vi "Main.vi"() -> ()   [LabVIEW 2017]
uses:
  type defs/states.ctl
  <vilib>/myRIO/Express VI/Onboard Devices/LED/LED Express VI.xnode
  <vilib>/myRIO/Instrument Drivers/Onboard IO/DIO/vis/Write.vi
  <vilib>/myRIO/Instrument Drivers/Onboard IO/DIO/DIO.lvlib
  <vilib>/myRIO/Common/Instrument Driver Framework/myRIO v1.0/DIO/typedefs/DIO Channels Enum.ctl
  <vilib>/myRIO/Common/Instrument Driver Framework/myRIO v1.0/DIO/typedefs/DIO Channels List.ctl
  <vilib>/myRIO/Common/Instrument Driver Framework/Utilities/typedefs/Generic FPGA Reference.ctl
  <vilib>/myRIO/Common/Instrument Driver Framework/Utilities/typedefs/myRIO v1.0 Reference.ctl
  <vilib>/myRIO/Common/Instrument Driver Framework/Utilities/typedefs/Hardware Version Enum.ctl
  <vilib>/myRIO/Common/Instrument Driver Framework/Utilities/typedefs/myRIO Generic Hardware Reference.ctl
  <vilib>/myRIO/Instrument Drivers/Onboard IO/DIO/typedefs/DIO Reference.ctl
  <vilib>/myRIO/Instrument Drivers/Onboard IO/DIO/vis/myRIO DIO Open.xnode
  <vilib>/myRIO/Common/Instrument Driver Framework/Utilities/vis/Is FPGA Ref Available.vi
  <vilib>/myRIO/Common/Instrument Driver Framework/myRIO v1.0/DIO/vis/myRIO v1.1 Open DIO.vi
  <vilib>/userdefined/High Color/nirio_resource_hc.ctl
  <vilib>/myRIO/Express VI/Onboard Devices/Button/Button Express VI.xnode
  type defs/task.ctl
  <vilib>/myRIO/Instrument Drivers/Onboard IO/PWM/typedefs/PWM Configuration.ctl
  <vilib>/myRIO/Instrument Drivers/Onboard IO/PWM/PWM.lvlib
  <vilib>/myRIO/Common/Instrument Driver Framework/myRIO v1.0/PWM/typedefs/PWM Channels Enum.ctl
  <vilib>/myRIO/Instrument Drivers/Onboard IO/PWM/typedefs/PWM Reference.ctl
  <vilib>/myRIO/Common/Instrument Driver Framework/myRIO v1.0/PWM/vis/myRIO v1.1 Open PWM.vi
  <vilib>/myRIO/Instrument Drivers/Onboard IO/PWM/vis/myRIO PWM Open.xnode
  <vilib>/myRIO/Express VI/Onboard IO/PWM/PWM Express VI.xnode
  <vilib>/myRIO/Express VI/Onboard IO/DO/DO Express VI.xnode
  <vilib>/myRIO/Instrument Drivers/Utilities/Utilities.lvlib
  type defs/data.ctl
  <vilib>/vision/Image Controls.llb/IMAQ Image.ctl
  <vilib>/vision/NI_Vision_Development_Module.lvlib
  <vilib>/myRIO/Instrument Drivers/Onboard IO/I2C/I2C.lvlib
  <vilib>/myRIO/Instrument Drivers/Onboard IO/Encoder/Encoder.lvlib
  <vilib>/myRIO/Common/Instrument Driver Framework/myRIO v1.0/Encoder/typedefs/Encoder Signal Mode.ctl
  type defs/action buttons.ctl
  <vilib>/vision/driver/NI_Vision_Acquisition_Software.lvlib
  <vilib>/userdefined/High Color/IMAQdx.ctl
  <vilib>/myRIO/Instrument Drivers/Onboard IO/I2C/vis/myRIO I2C Open.xnode
  <vilib>/myRIO/Instrument Drivers/Onboard IO/I2C/typedefs/I2C Reference.ctl
  <vilib>/myRIO/Instrument Drivers/Onboard IO/I2C/typedefs/I2C Configuration.ctl
  <vilib>/myRIO/Instrument Drivers/Onboard IO/I2C/typedefs/I2C Transfer Rate.ctl
  <vilib>/myRIO/Common/Instrument Driver Framework/myRIO v1.0/I2C/typedefs/I2C Channels Enum.ctl
  <vilib>/myRIO/Common/Instrument Driver Framework/myRIO v1.0/I2C/vis/myRIO v1.1 Open I2C.vi
  type defs/mode buttons.ctl
  <vilib>/vision/Pattern Matching.llb/IMAQ GM Match Report.ctl
panel:
  out "State":T1(ring)
  in  "BackStates":enum16{"0", "1", "2", "3", "4", "5", "6", ""}(ring)
  in  "At Def pos":bool
  out "Grabbed":bool
  in  "error in":errorcluster
  out "error out 4":errorcluster
  out "error out 3":errorcluster
  out "error out 2":errorcluster
  in  "Def PWM":dbl=0.5
  out "Found Right Ball":bool=TRUE
  out "FT_G_enc":i32[](array[numeric])
  out "FT_M_enc":i32[](array[numeric])
  out "FT_Right_enc":i32[](array[numeric])
  out "FT_Left_enc":i32[](array[numeric])
  out "FT_Angles":dbl[](array[numeric])
  out "Dots of States":i32[][](array[numeric])
  in  "States in total":i32
  in  "(auto) States":T2(ring)
  out "G_enc":i32[](array[numeric])
  out "M_enc":i32[](array[numeric])
  out "Right_enc":i32[](array[numeric])
  out "Left_enc":i32[](array[numeric])
  out "Angles":dbl[](array[numeric])
  in  "Dots in total":i32
  in  "CurDot":T3(ring)
  out "(auto) balls counter":i32
  out "distance to the side":u32
  out "value Z 2":ext
  out "value Z":ext
  in  ",ctl num":i32
  in  ".Task":enum16{"Def", "<mod>[P]+tnl ", "(auto)"}(ring)
  out "Pattern classes":i32[](array[numeric])
  in  "5":i32
  in  "4":i32
  in  "3":i32
  in  "1":i32
  in  "2":i32
  out "5b":bool
  out "4b":bool
  out "3b":bool
  out "2b":bool
  out "1b":bool
  out "Color classes":i32[](array[numeric])
  in  "Next step":bool
  in  "ball = pattern?":bool
  out "error out":errorcluster
  in  "Tab Control":enum32{"Motors", "Ball", "Pattern", "Camera"}(tab)
  in  "Left+":bool
  in  "Left-":bool
  in  "Right+":bool
  in  "Right-":bool
  in  "G-":bool
  in  "G+":bool
  in  "M+":bool
  in  "M-":bool
  in  "M_PWM":dbl=0.4
  in  "L_PWM":dbl=0.5
  in  "R_PWM":dbl=0.5
  in  "Reset M_enc":bool
  out "M_enc_value":i32
  in  "Reset G_enc":bool
  out "G_enc_value":i32
  in  "G_PWM":dbl=0.4
  in  "M_UB_Align":i32=-800
  in  "G_UB_Align":i32
  in  "M_UB_grab":i32=-800
  in  "G_UB_grab":i32=-500
  in  "Manip state":enum16{"Align", "Grab", "Release", "PickUp"}(ring)
  in  "Reset L_enc":bool
  out "L_enc_value":i32
  in  "Reset R_enc":bool
  out "R_enc_value":i32
  in  "G_UB_pickUp":i32
  in  "M_UB_pickUp":i32
  in  "Balls to remember":i32
  out "Circles Calibrated (Shape Detection 1)":T4(array[cluster]) {"Position"."Y" format="%.2f"; "Position"."X" format="%.2f"}
  out "Number of Matches (Shape Detection 1)":i32
  out "Color":i32
  in  "Align X - t, Y - f":bool
  out "CircleRadius":dbl
  in  "defX":dbl=360.0
  in  "RangeY":dbl=30.0
  in  "defY":dbl=380.0
  out "X is in range":bool
  out "Y is in range":bool
  out "curX":dbl
  out "curY":dbl
  out "1y1 (circle)":i32
  out "1x1 (circle)":i32
  out "1x0 (circle)":i32
  out "1y0 (circle)":i32
  in  "divider (circle)":dbl=1.0
  in  "ROI Descriptor COLOR":T5={"Global Rectangle"=[86, 71, 180, 164], "Contours"=[{"ID"=enum."External", "Type"=3, "Coordinates"=[86, 71, 180, 164]}]} {"Contours"."Type" items=["No Selection", "Point", "Line", "Rectangle", "Oval", "Polygon", "Freehand Region", "Annulus", "Unused2", "Unused3", "Broken Line", "Freehand Line", "Rotated Rectangle"]}
  in  "align accuracy":u32=100
  in  "Ball number":i32=1
  out "ball match":bool
  in  "RangeX":dbl=40.0
  out "Ready to Grab":bool
  in  "Range(p)":sgl=30.0
  in  "defX(p)":sgl=320.0
  out "Pattern":i32
  out "y0":i32
  out "x0":i32
  out "x1":i32
  out "y1":i32
  out "Number of Matches (Geometric Matching 1)":i32
  out "Calibrated Matches (Geometric Matching 1)":T6[](array[typedef]) {"Correlation Score" format="%.2f"; "Target Template Curve Score" format="%.2f"; "Template Target Curve Score" format="%.2f"; "Bounding Box"."y" format="%.2f"; "Bounding Box"."x" format="%.2f"; "Position"."y" format="%.2f"; "Position"."x" format="%.2f"; "Score" format="%.2f"; "Scale" format="%.2f"; "Angle" format="%.2f"; "Occlusion %" format="%.2f"}
  out "Scale":sgl
  in  "divider (pattern)":sgl=1.0
  out "curX(p)":sgl
  out "In Range? (p)":bool
  in  "align accuracy (p)":u32=100
  in  "patterns to remember":i32=3
  out "pattern match":bool
  in  "M duty cycle [P]":dbl=990.0 format="%#_13g"
  in  "S duty cycle [P]":dbl=990.0 format="%#_13g"
  in  "S duty cycle [B]":dbl=500.0 format="%#_13g"
  in  "M duty cycle [B]":dbl=720.0 format="%#_13g"
  in  "S duty cycle [F]":dbl=620.0 format="%#_13g"
  in  "M duty cycle [F]":dbl=620.0 format="%#_13g"
  in  "Angle for pattern (degrees)":sgl=90.0 format="%.2f"
  out "rotate":bool=TRUE
  in  "PWM channel (m)":tag="B/PWM2"
  in  "[cur] duty cycle [%] (m)":dbl
  in  "PWM channel (s)":tag="A/PWM2"
  in  "[cur] duty cycle [%] (s)":dbl
  in  "Camera state":enum16{"Fwd", "Pattern", "Ball"}(ring)
  in  "Angle for Align (degrees)":sgl=2.0 format="%.2f"
  in  "mode buttons":T7
  out "image display":T8(plugin-control)
  in  "action buttons":T9
  in  "Stop":bool
  # "Machine\nVision\nApp"
  # "less = slower"
  # "less = slower"
  # "0 - 640x480"
  # "5 - 1280x720"
  # "30 - 320x240"
  # "35 - 800x600"
  # "40 - 176x144"
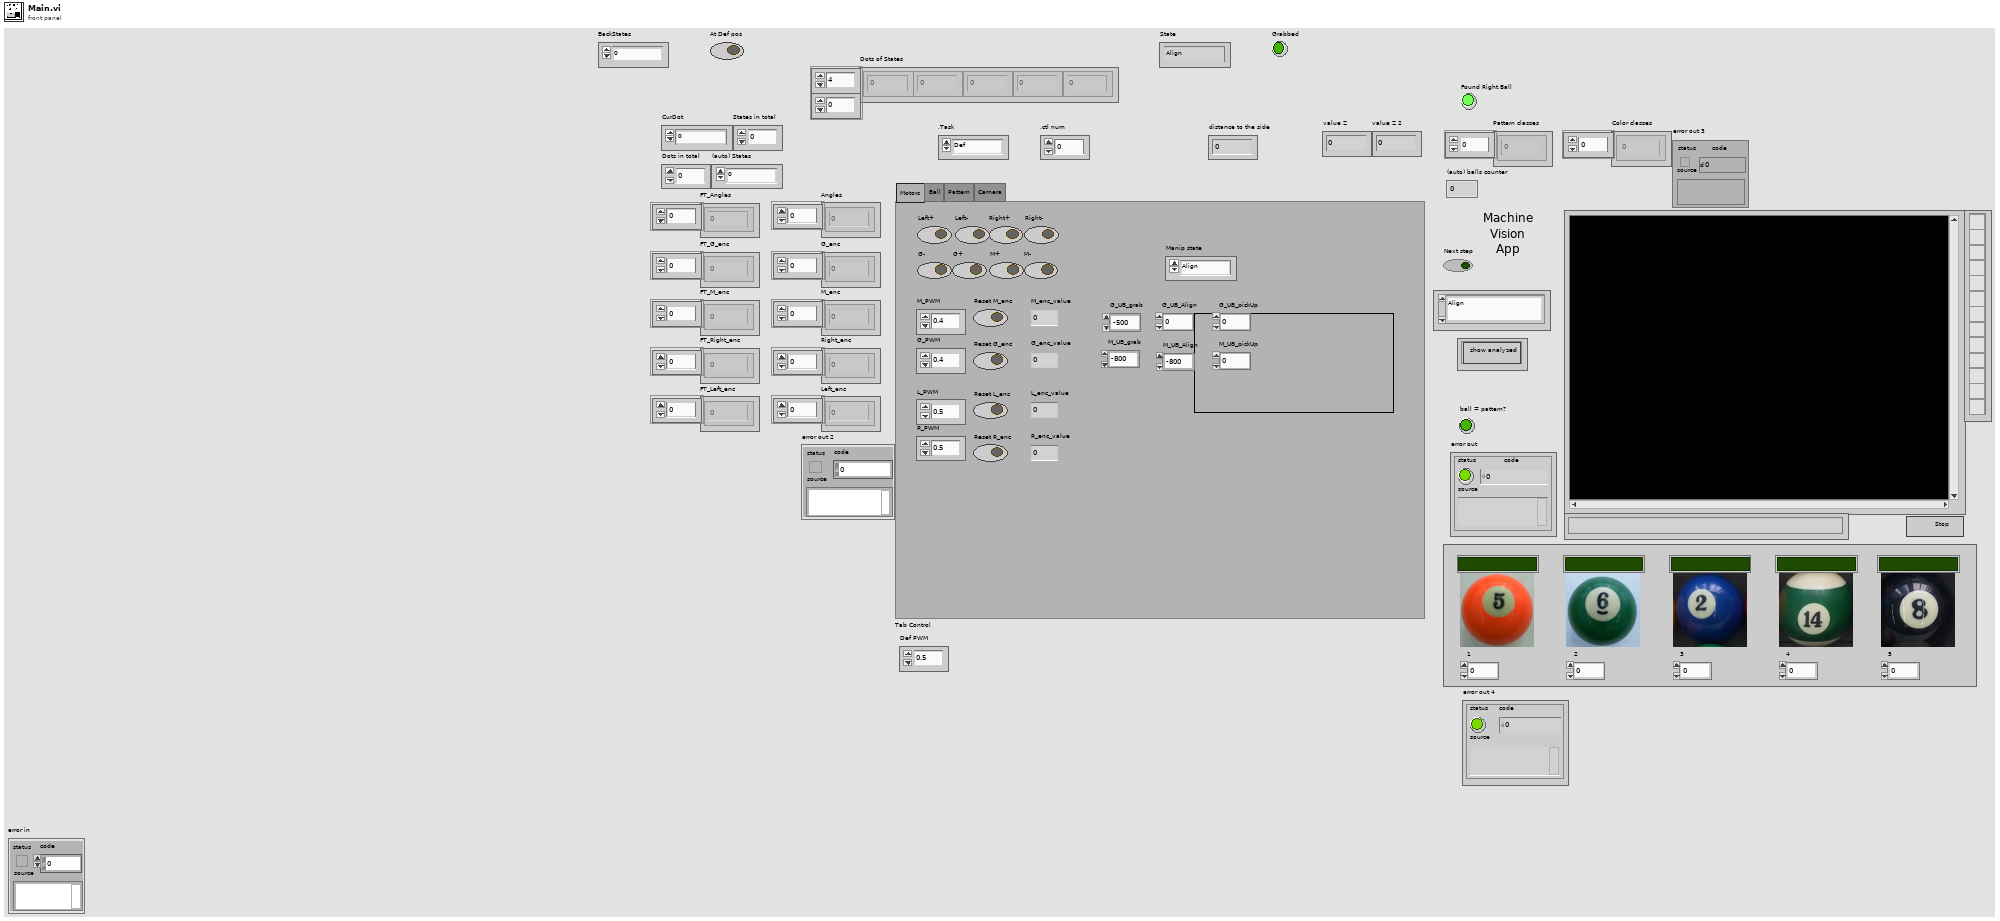
[diagram p1: front panel]
types:
  T1 = enum16{"Align", "1", "2", "3", "4", "5", "6", "7", "8", "9", "10", "11", "12", "13", "(pattern) Align", "Pattern", "(mod) pattern", "<mod>[P] remembering", "<mod>[P] go through tunnel", "<mod>[P] comparing", "(mod) ball", "Ball", "Other", "Clear", "navx", "(auto) Balls Analyze", "(auto) Ball Analyze", "(pattern) Align <loop>", "(ball) Align <loop>", "(auto) Recover Def Pos", "(auto) Go Back", "Joystick control"}
  T2 = enum16{"0", "1", "2", "3", "4", "5", "6", "7", "8", "9", "10"}
  T3 = enum16{"0", "1", "2", "3", "4", "5", "6", "7", "8", "9", "10", "11", "12", "13", "14", "15", "16", "17", "18", "19", "20", "21", "22", "23", "24", "25", "26", "27", "28", "29", "30", "31", "32", "33", "34", "35"}
  T4 = cluster{"Position":cluster{"X":sgl, "Y":sgl}, "Radius":dbl, "Score":dbl}[]
  T5 = cluster{"Global Rectangle":i32[], "Contours":cluster{"ID":enum32{"External", "Internal"}, "Type":u32, "Coordinates":i32[]}[]}
  T6 = typedef "IMAQ GM Match Report.ctl" = cluster{"Position":cluster{"x":sgl, "y":sgl}, "Angle":sgl, "Scale":sgl, "Score":sgl, "Bounding Box":cluster{"x":sgl, "y":sgl}[], "Contrast Reversed":bool, "Occlusion %":sgl, "Template Target Curve Score":sgl, "Target Template Curve Score":sgl, "Correlation Score":sgl}
  T7 = typedef "mode buttons.ctl" = cluster{"show analyzed":bool}
  T8 = typedef "IMAQ Image.ctl" = refnum<image>
  T9 = typedef "action buttons.ctl" = cluster{"State":enum16{"Align", "1", "2", "3", "4", "5", "6", "7", "8", "9", "10", "11", "12", "13", "(pattern) Align", "Pattern", "(mod) pattern", "<mod>[P] remembering", "<mod>[P] go through tunnel", "<mod>[P] comparing", "(mod) ball", "Ball", "Other", "Clear", "navx", "(auto) Balls Analyze", "(auto) Ball Analyze", "(pattern) Align <loop>", "(ball) Align <loop>", "(auto) Recover Def Pos", "(auto) Go Back", "Joystick control"}}
  T10 = typedef "Encoder Signal Mode.ctl" = enum16{"Quadrature phase signal", "Step and direction signal"}
  T11 = typedef "data.ctl" = cluster{"Shape - t, Color - f":bool, "qsm":cluster{"Webcam image ref":T8, "Analyzed image ref":T8, "Stop webcam":bool}, " image ref":T8, "number img":i32, "ROI Descriptor (Image Mask 1)":cluster{"Global Rectangle":i32[], "Contours":cluster{"ID":enum32{"External", "Internal"}, "Type":u32, "Coordinates":i32[]}[]}, "Pattern class":i32, "Color class":i32, "Color classes":i32[], "Pattern classes":i32[], "Session Out":T12}
  T12 = typedef "IMAQdx.ctl" = refnum<k21>
  T13 = typedef "states.ctl" = enum16{"(qsm) schedule", "(qsm) initialize", "(qsm) release", "(qsm) clean up", "(qsm) shutdown", "(myRIO) initialize", "(myRIO) clean up", "(myRIO) update ports", "Setup get", "(image) get", "(image) show", "(ball) Shape detection", "(ball) Calc ball indx", "(ball) Calculate ROI", "(ball) Analyze color", "(ball) Align", "(ball) Wait", "(ball) Grab", "(pattern) Find Square", "(pattern) Calculate ROI", "(pattern) Calc pattern indx", "Compare", "(pattern) Analyze pattern", "(pattern) Align", "(pattern) Wait", "(pattern) states control", "navx", "stop motors", "(joystick) Joystick control", "_Timer", "Setup manipulator", "(auto) Count balls", "(auto) Analyze balls", "(auto) Dot Controller", "(auto) Fwd (cm)", "(auto) Turn (angle)", "(auto) Tnl (M2-M2.5)", "(auto) Recover Def Pos", "(auto) Go Back Controller", "Wait for button"}
  T14 = typedef "Encoder.lvlib/Encoder Reference.ctl" = cluster{"myRIO Reference":T15, "Encoder Channels Enum":T19}
  T15 = typedef "myRIO Generic Hardware Reference.ctl" = cluster{"myRIO Model":T16, "myRIO Hardware Reference":T17}
  T16 = typedef "Hardware Version Enum.ctl" = enum16{"Unknown", "myRIO-1900", "myRIO-1950", "roboRIO", "NI ELVIS RIO CM"}
  T17 = typedef "myRIO v1.0 Reference.ctl" = cluster{"Generic FPGA Reference":T18, "Allow multiple opens":bool}
  T18 = typedef "Generic FPGA Reference.ctl" = refnum<k20>
  T19 = typedef "Encoder Channels Enum.ctl" = enum16{"Not Connected", "C/ENC0", "C/ENC1", "A/ENC", "B/ENC", "DIO/ENC0", "DIO/ENC1", "DIO/ENC2", "DIO/ENC3", "DIO/ENC4"}
  T20 = typedef "PWM.lvlib/PWM Reference.ctl" = cluster{"myRIO Reference":T15, "PWM Channels Enum":T21, "PWM Configuration":T22}
  T21 = typedef "PWM Channels Enum.ctl" = enum16{"Not Connected", "C/PWM0", "C/PWM1", "A/PWM0", "A/PWM1", "A/PWM2", "B/PWM0", "B/PWM1", "B/PWM2", "PWM/PWM0", "PWM/PWM1", "PWM/PWM2", "PWM/PWM3", "PWM/PWM4", "PWM/PWM5", "PWM/PWM6", "PWM/PWM7", "PWM/PWM8", "PWM/PWM9"}
  T22 = typedef "PWM.lvlib/PWM Configuration.ctl" = cluster{"Frequency":dbl, "Duty Cycle":dbl}
  T23 = typedef "I2C.lvlib/I2C Reference.ctl" = cluster{"myRIO Reference":T15, "I2C Channels Enum":T24, "I2C Configuration":T25}
  T24 = typedef "I2C Channels Enum.ctl" = enum16{"Not Connected", "A/I2C", "B/I2C", "I2C/I2C"}
  T25 = typedef "I2C.lvlib/I2C Configuration.ctl" = cluster{"I2C Transfer Rate":T26}
  T26 = typedef "I2C.lvlib/I2C Transfer Rate.ctl" = enum16{"Standard mode (100 kbps)", "Fast mode (400 kbps)"}
  T27 = typedef "nirio_resource_hc.ctl" = tag
  T28 = typedef "DIO.lvlib/DIO Reference.ctl" = cluster{"myRIO Reference":T15, "DIO Channels List":T29}
  T29 = typedef "DIO Channels List.ctl" = T30[]
  T30 = typedef "DIO Channels Enum.ctl" = enum16{"Not Connected", "C/DIO0", "C/DIO1", "C/DIO2", "C/DIO3", "C/DIO4", "C/DIO5", "C/DIO6", "C/DIO7", "A/DIO0", "A/DIO1", "A/DIO2", "A/DIO3", "A/DIO4", "A/DIO5", "A/DIO6", "A/DIO7", "A/DIO8", "A/DIO9", "A/DIO10", "A/DIO11", "A/DIO12", "A/DIO13", "A/DIO14", "A/DIO15", "B/DIO0", "B/DIO1", "B/DIO2", "B/DIO3", "B/DIO4", "B/DIO5", "B/DIO6", "B/DIO7", "B/DIO8", "B/DIO9", "B/DIO10", "B/DIO11", "B/DIO12", "B/DIO13", "B/DIO14", "B/DIO15", "LED0", "LED1", "LED2", "LED3", "Button0", "DIO/DIO0", "DIO/DIO1", "DIO/DIO2", "DIO/DIO3", "DIO/DIO4", "DIO/DIO5", "DIO/DIO6", "DIO/DIO7", "DIO/DIO8", "DIO/DIO9", "SPI/CS0", "SPI/CS1", "SPI/CS2", "SPI/CS3", "LED RADIO (Green)", "LED RADIO (Red)", "LED COMM (Green)", "LED COMM (Red)", "LED MODE (Green)", "LED MODE (Red)"}
  T31 = enum16{"Align", "(pattern) Align", "Pattern", "(mod) pattern", "(mod) ball", "Ball", "Other", "Clear", "Joystick control"}
  T32 = enum16{"Align", "(pattern) Align", "Pattern", "(mod) pattern", "<mod>[P] remembering", "<mod>[P] go through tunnel", "<mod>[P] comparing", "(mod) ball", "Ball", "Other", "Clear", "Joystick control"}
  T33 = enum16{"Align", "(pattern) Align", "Pattern", "(mod) pattern", "<mod>[P]+move", "(mod) ball", "Ball", "Other", "Clear", "Joystick control"}
  T34 = typedef "task.ctl" = T13[]
  T35 = typedef "Image Type" = u32
  T36 = cluster{"Position":cluster{"X":sgl, "Y":sgl}, "Radius":dbl, "Score":dbl}
  T37 = cluster{"Webcam image ref":T8, "Analyzed image ref":T8, "Stop webcam":bool}
  T38 = cluster{"ID":enum32{"External", "Internal"}, "Type":u32, "Coordinates":i32[]}[]
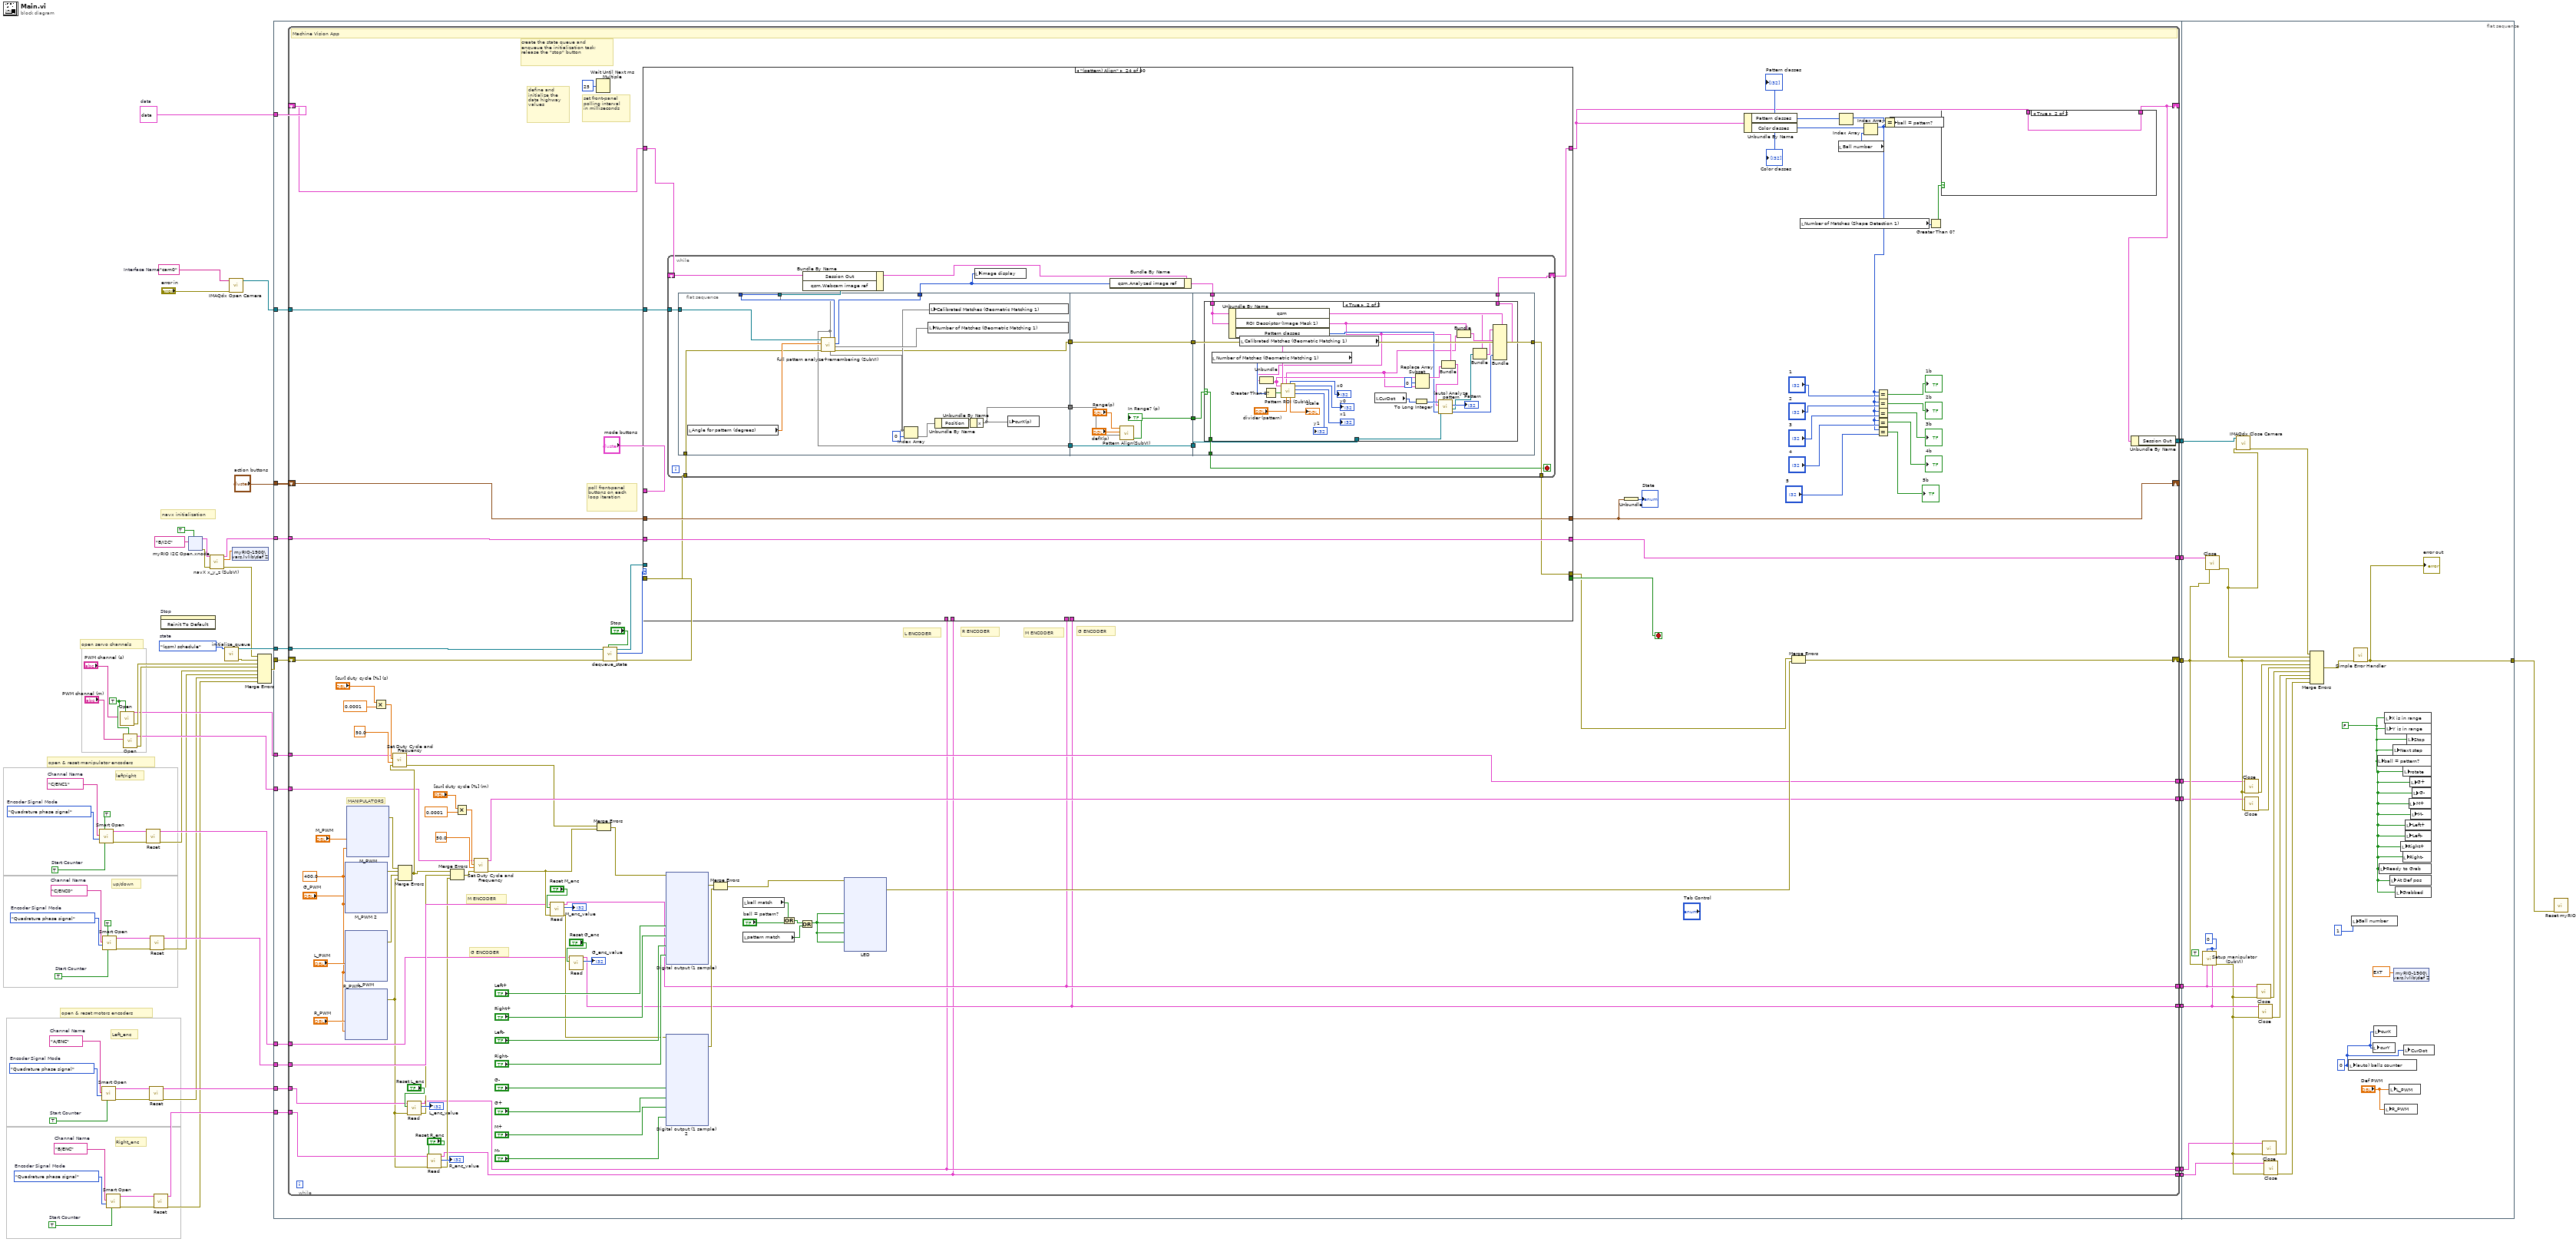
[diagram p0: block diagram]
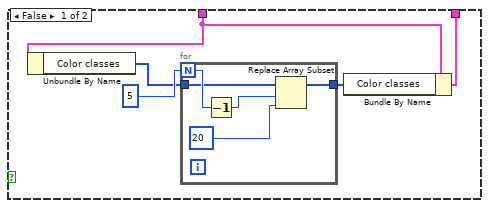
[diagram p2: hidden frame]
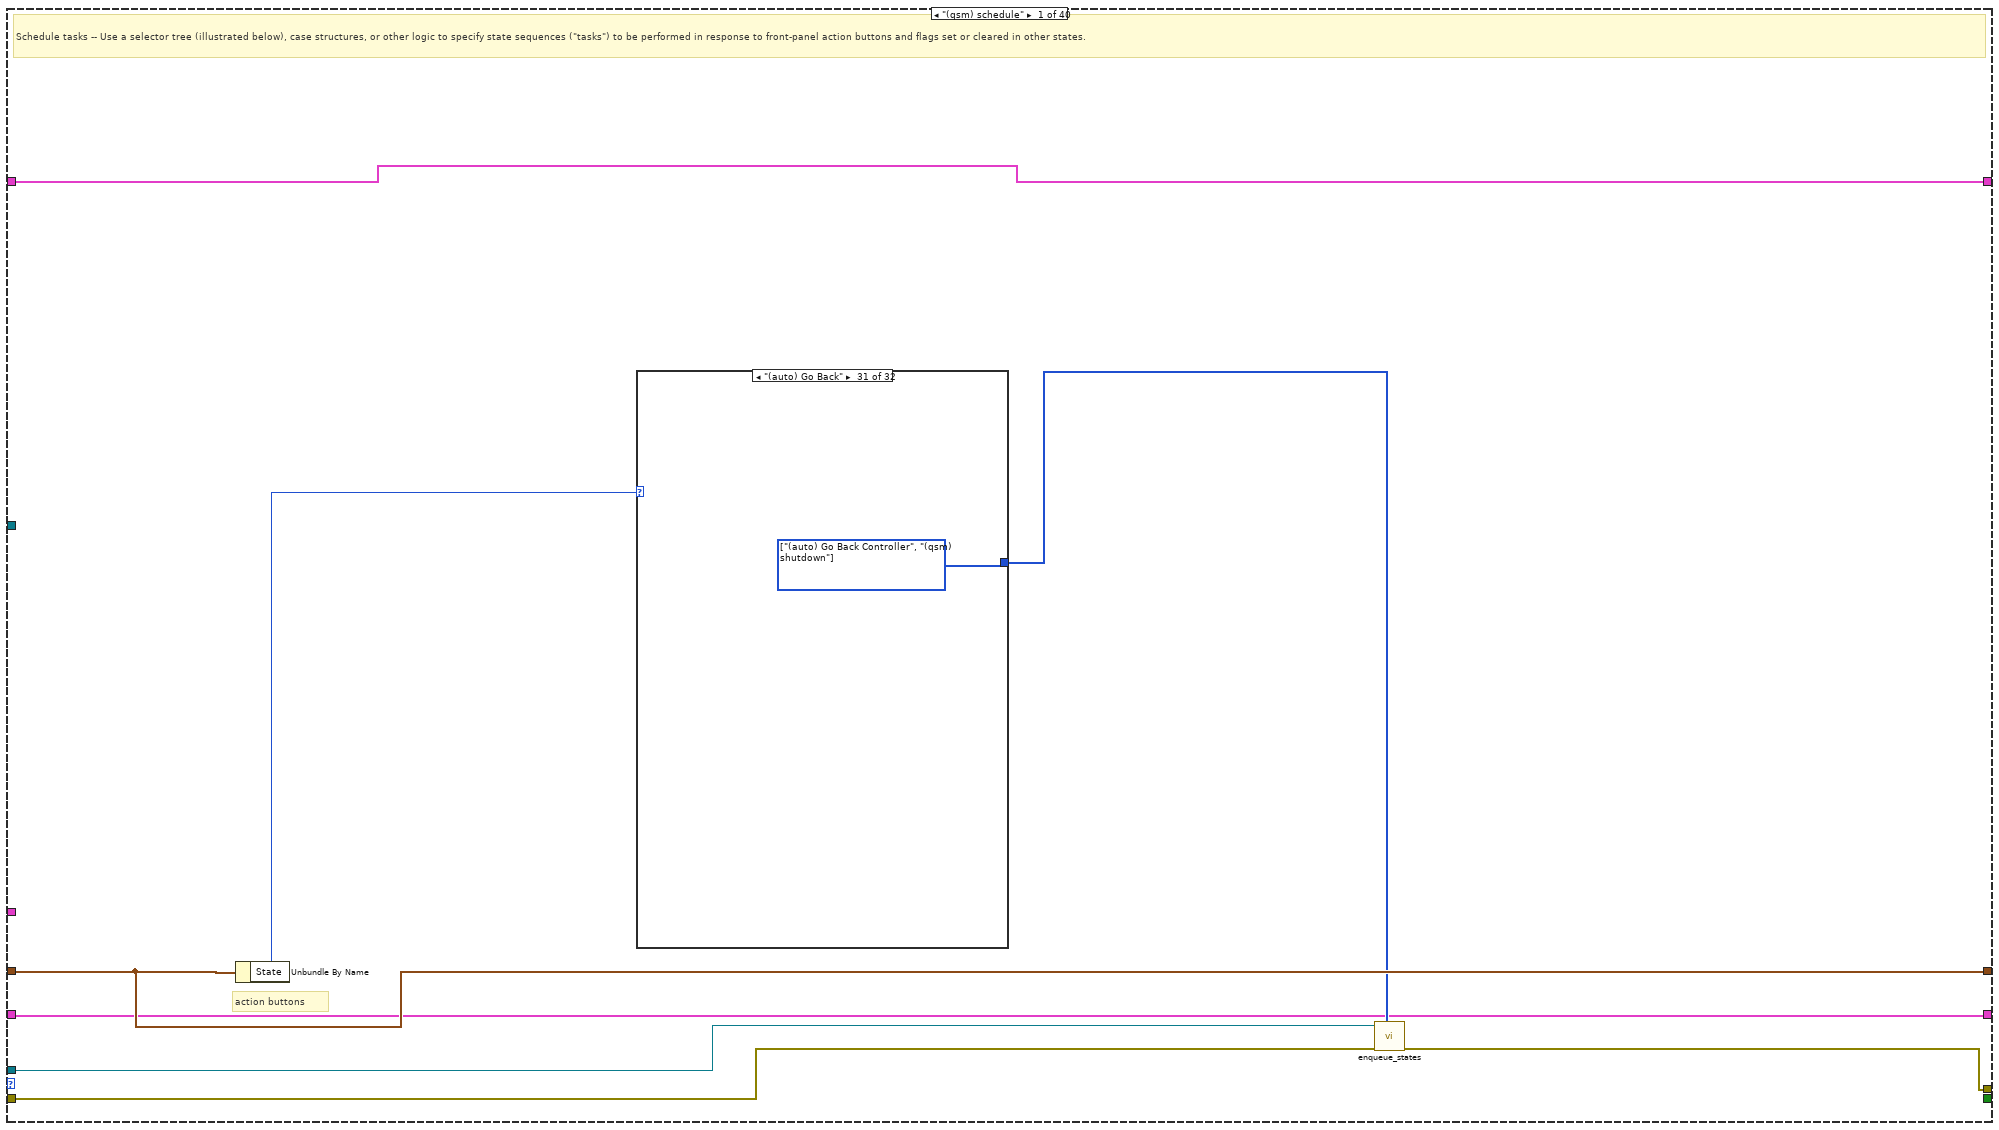
[diagram p3: hidden frame]
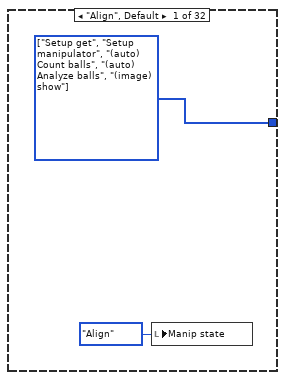
[diagram p4: hidden frame]
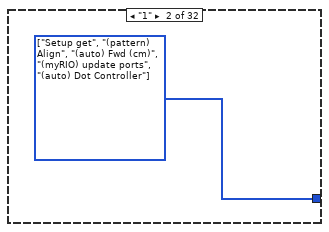
[diagram p5: hidden frame]
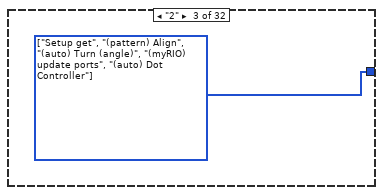
[diagram p6: hidden frame]
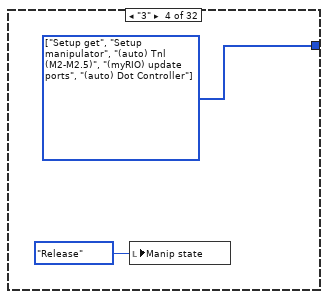
[diagram p7: hidden frame]
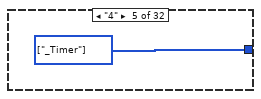
[diagram p8: hidden frame]
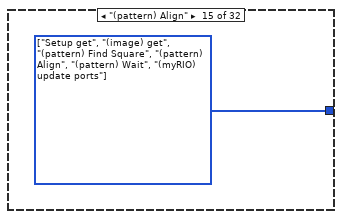
[diagram p18: hidden frame]
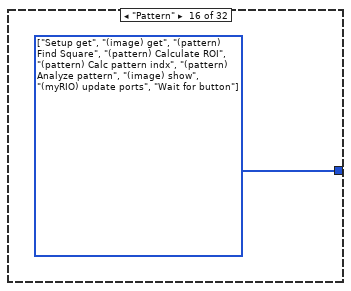
[diagram p19: hidden frame]
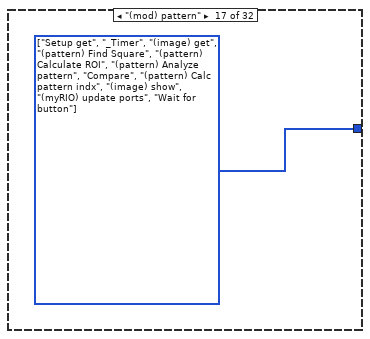
[diagram p20: hidden frame]
diagram:
  w10 = "cam0"  # Interface Name
  w19 = TRUE  # Start Counter
  w18 = TRUE  # Start Counter
  w22 = Encoder_Signal_Mode."Quadrature phase signal"  # Encoder Signal Mode
  w23 = tag "B/ENC"  # Channel Name
  w26 = Encoder_Signal_Mode."Quadrature phase signal"  # Encoder Signal Mode
  w27 = tag "A/ENC"  # Channel Name
  w35 = TRUE  # Start Counter
  w36 = Encoder_Signal_Mode."Quadrature phase signal"  # Encoder Signal Mode
  w37 = tag "C/ENC1"  # Channel Name
  w41 = TRUE  # Start Counter
  w42 = Encoder_Signal_Mode."Quadrature phase signal"  # Encoder Signal Mode
  w43 = tag "C/ENC0"  # Channel Name
  w50 = TRUE ("Allow multiple opens?")
  w47 = T11 {"Shape - t, Color - f"=FALSE, "qsm"={"Webcam image ref"=refnum, "Analyzed image ref"=refnum, "Stop webcam"=FALSE}, " image ref"=refnum, "number img"=0, "ROI Descriptor (Image Mask 1)"={"Global Rectangle"=[109, 72, 345, 284], "Contours"=[{"ID"=enum."External", "Type"=3, "Coordinates"=[109, 72, 345, 284]}]}, "Pattern class"=0, "Color class"=0, "Color classes"=[], "Pattern classes"=[], "Session Out"=""}  # data
  w58 = states."(qsm) schedule"  # state
  # "navx initialization"
  # "open & reset motors encoders"
  # "Right_enc"
  # "Left_enc"
  # "left/right"
  # "up/down"
  # "open servo channels"
  # "open & reset manipulator encoders"
  n1 = call <vilib>:"Smart Open.vi"("Start Counter"=w35, "Allow multiple opens?"=TRUE, "Encoder Signal Mode"=w36, "Channel Name"=w37) -> ("error out"=w33:errorcluster, "Encoder Ref Out"=w34:T14)  [unwired: 6 in]
  n2 = call <vilib>:"Smart Open.vi"("Start Counter"=w18, "Encoder Signal Mode"=w26, "Channel Name"=w27) -> ("error out"=w24:errorcluster, "Encoder Ref Out"=w25:T14)  [unwired: 7 in]
  n3 = call <vilib>:"Smart Open.vi"("Start Counter"=w41, "Allow multiple opens?"=TRUE, "Encoder Signal Mode"=w42, "Channel Name"=w43) -> ("error out"=w39:errorcluster, "Encoder Ref Out"=w40:T14)  [unwired: 6 in]
  n4 = call <vilib>:"Smart Open.vi"("Start Counter"=w19, "Encoder Signal Mode"=w22, "Channel Name"=w23) -> ("error out"=w20:errorcluster, "Encoder Ref Out"=w21:T14)  [unwired: 7 in]
  n5 = call <vilib>:"Open.vi"("Allow multiple opens?"=w50, "Channel Name"="PWM channel (s)") -> ("error out"=w56:errorcluster, "PWM Ref Out"=w54:T20)  [unwired: 8 in]
  n6 = call <vilib>:"Open.vi"("Allow multiple opens?"=w50, "Channel Name"="PWM channel (m)") -> ("error out"=w55:errorcluster, "PWM Ref Out"=w53:T20)  [unwired: 8 in]
  n7 = call <vilib>:"Reset.vi"("error in (no error)"=w33, "Encoder Ref In"=w34) -> ("error out"=w28:errorcluster, "Encoder Ref Out"=w32:T14)  [unwired: 8 in]
  n8 = call <vilib>:"Reset.vi"("error in (no error)"=w24, "Encoder Ref In"=w25) -> ("error out"=w15:errorcluster, "Encoder Ref Out"=w17:T14)  [unwired: 8 in]
  n9 = call <vilib>:"Reset.vi"("error in (no error)"=w39, "Encoder Ref In"=w40) -> ("error out"=w29:errorcluster, "Encoder Ref Out"=w38:T14)  [unwired: 8 in]
  n10 = call <vilib>:"Reset.vi"("error in (no error)"=w20, "Encoder Ref In"=w21) -> ("error out"=w14:errorcluster, "Encoder Ref Out"=w16:T14)  [unwired: 8 in]
  n11 = invoke on="Stop" class="Bool (strict)" method="Reinit To Default"() -> ()  [unwired: 3 in, 3 out]
  n12 = xnode "myRIO I2C Open.xnode"("Allow multiple opens?"=TRUE, "Channel Name"=tag "B/I2C") -> ("error out"=w4:errorcluster, "I2C Ref Out"=w5:T23)  [unwired: 1 in]
  n13 = call "navX x_y_z (SubVI).vi"("I2C Ref Out in"=w5, "error in (no error)"=w4) -> ("I2C Ref Out out"=w44:T23, "value Z"=w6:ext, "error out"=w45:errorcluster)  [unwired: 9 in, 2 out]
  n14 = call "initialize_queue.vi"("state"=w58) -> ("error out"=w59:errorcluster, "queue out"=w60:refnum<queue>)  [unwired: 9 in]
  n15 = call <vilib>:"IMAQdx Open Camera.vi"("error in"="error in", "Session In"=w10) -> ("Session Out"=w9:T12)  [unwired: 1 in, 8 out]
  n16 = shared-variable "myRIO-1900\\vars.lvlib\\def Z"(w6) -> ()  [unwired: 1 in, 1 out]
  n17 = Merge Errors(w45, w59, w56, w55, w28, w29, w15, w14) -> (w57:errorcluster)
  n18 = flat-sequence {
    tunnel: [w84] -> w62
    tunnel: "action buttons" -> [w83]
    tunnel: w57 -> [w81]
    tunnel: w60 -> [w82]
    tunnel: w47 -> [w80]
    tunnel: w54 -> [w79]
    tunnel: w53 -> [w78]
    tunnel: [w77] -> w52
    tunnel: [w76] -> w51
    tunnel: w44 -> [w75]
    tunnel: [w74] -> w46
    tunnel: w38 -> [w73]
    tunnel: w32 -> [w72]
    tunnel: [w71] -> w31
    tunnel: [w70] -> w30
    tunnel: w17 -> [w69]
    tunnel: w16 -> [w68]
    tunnel: [w67] -> w13
    tunnel: [w66] -> w12
    tunnel: w9 -> [w65]
    tunnel: [w64] -> w8
    tunnel: [w1437] -> w63
    tunnel: w62 -> [w1428]
    tunnel: w52 -> [w1426]
    tunnel: w51 -> [w1425]
    tunnel: w46 -> [w1432]
    tunnel: w31 -> [w1423]
    tunnel: w30 -> [w1424]
    tunnel: w13 -> [w1420]
    tunnel: w12 -> [w1421]
    tunnel: w8 -> [w1414]
    frame #0 {
      n19 = while {
        shift-right: [w179] -> w84
        shift-left: w81 -> [w184]
        shift-right: [w87] -> _
        shift-left: w80 -> [w89]
        shift-right: [w91] -> _
        shift-left: w83 -> [w168]
        tunnel: w82 -> [w167]
        tunnel: w79 -> [w130]
        tunnel: w78 -> [w114]
        tunnel: [w127] -> w77
        tunnel: [w126] -> w76
        tunnel: w75 -> [w124]
        tunnel: [w123] -> w74
        tunnel: w73 -> [w116]
        tunnel: w72 -> [w115]
        tunnel: [w112] -> w71
        tunnel: [w113] -> w70
        tunnel: w69 -> [w99]
        tunnel: w68 -> [w98]
        tunnel: [w93] -> w67
        tunnel: [w92] -> w66
        tunnel: w65 -> [w88]
        tunnel: [w86] -> w64
        stop <- w166 stop-if-true
        w105 = 400.0 ("Frequency [Hz]")
        # "R ENCODER"
        # "L ENCODER"
        # "G ENCODER"
        # "M ENCODER"
        # "G ENCODER"
        # "M ENCODER"
        # "define and \ninitialize the \ndata highway\nvalues"
        # "MANIPULATORS"
        # "create the state queue and\nenqueue the initialization task;\nrelease the \"stop\" button"
        # "set front-panel\npolling interval\nin milliseconds"
        # "poll front-panel\nbuttons on each\nloop iteration"
        # "Machine Vision App"
        n20 = xnode "M_PWM 2"("Duty Cycle"="G_PWM", "Frequency [Hz]"=w105) -> ("error out"=w106:errorcluster)  [unwired: 1 in]
        n21 = xnode "L_PWM"("Duty Cycle"="L_PWM", "Frequency [Hz]"=w105) -> ("error out"=w178:errorcluster)  [unwired: 1 in]
        n22 = xnode "R_PWM"("Duty Cycle"="R_PWM", "Frequency [Hz]"=w105) -> ("error out"=w97:errorcluster)  [unwired: 1 in]
        n23 = xnode "M_PWM"("Duty Cycle"="M_PWM", "Frequency [Hz]"=w105) -> ("error out"=w107:errorcluster)  [unwired: 1 in]
        n24 = Multiply(x="[cur] duty cycle [%] (s)", y=0.0001) -> (x*y=w133:dbl)
        n25 = Merge Errors(w107, w106, w178, w97) -> (w129:errorcluster)
        n26 = call <vilib>:"Set Duty Cycle and Frequency.vi"("error in (no error)"=w129, "Frequency [Hz]"=50.0 ("freq [Hz]"), "Duty Cycle"=w133, "PWM Ref In"=w130) -> ("error out"=w125:errorcluster, "PWM Ref Out"=w127:T20)  [unwired: 5 in]
        n27 = call <vilib>:"Read.vi"("error in (no error)"=w97, "Reset Counter"="Reset L_enc", "Encoder Ref In"=w99) -> ("error out"=w95:errorcluster, "Counter Value"=→"L_enc_value":i32, "Encoder Ref Out"=w93:T14)  [unwired: 4 in, 2 out]
        n28 = call <vilib>:"Read.vi"("error in (no error)"=w97, "Reset Counter"="Reset R_enc", "Encoder Ref In"=w98) -> ("error out"=w94:errorcluster, "Counter Value"=→"R_enc_value":i32, "Encoder Ref Out"=w92:T14)  [unwired: 4 in, 2 out]
        n29 = Merge Errors(w129, w95, w94) -> (w96:errorcluster)
        n30 = Multiply(x="[cur] duty cycle [%] (m)", y=0.0001) -> (x*y=w137:dbl)
        n31 = call <vilib>:"Set Duty Cycle and Frequency.vi"("error in (no error)"=w96, "Frequency [Hz]"=50.0 ("freq [Hz]"), "Duty Cycle"=w137, "PWM Ref In"=w114) -> ("error out"=w120:errorcluster, "PWM Ref Out"=w126:T20)  [unwired: 5 in]
        n32 = call <vilib>:"Read.vi"("error in (no error)"=w120, "Reset Counter"="Reset M_enc", "Encoder Ref In"=w116) -> ("error out"=w119:errorcluster, "Counter Value"=→"M_enc_value":i32, "Encoder Ref Out"=w113:T14)  [unwired: 4 in, 2 out]
        n33 = call <vilib>:"Read.vi"("Reset Counter"="Reset G_enc", "Encoder Ref In"=w115) -> ("Counter Value"=→"G_enc_value":i32, "Encoder Ref Out"=w112:T14)  [unwired: 5 in, 3 out]
        n34 = Wait Until Next ms Multiple(millisecond multiple=u32 25) -> ()  [unwired: 1 out]
        n35 = Merge Errors(w125, w120) -> (w128:errorcluster)
        n36 = call "dequeue_state.vi"("stop"="Stop", "error in (no error)"=w184, "queue in"=w167) -> ("error out"=w185:errorcluster, "state"=w180:T13, "queue out"=w169:refnum<queue>)  [unwired: 6 in]
        n37 = case shown="\"(pattern) Align\"" w180 {
          tunnel: w185 -> [w456 w502 w509 w513 w520 w529 w533 w580 w655 w695 w713 w730 w740 w757 w787 w800 w806 w837 w857 w863 w866 w870 w912 w917 w992 w1010 w1080 w1107 w1113 w1130 w1137 w1147 w1155 w1268 w1331 w1339 w1345 w1352 w1366 w1367]
          tunnel: w169 -> [w457 _ _ _ w527 _ _ _ _ _ _ _ _ _ _ _ w805 _ _ _ _ _ _ _ _ _ _ _ _ _ _ _ _ _ _ _ _ _ _ _]
          tunnel: [w451 w486 w509 w513 w519 w529 w532 w580 w655 w695 w713 w730 w740 w757 w787 w800 w806 w836 w857 w863 w866 w870 w912 w916 w992 w1010 w1080 w1107 w1113 w1130 w1137 w1147 w1173 w1268 w1332 w1338 w1344 w1351 w1366 w1367] -> w158
          tunnel: w168 -> [w455 w497 w511 w515 w523 w528 w535 w577 w658 w688 w715 w723 w745 w770 w795 w802 w808 w839 w846 w865 w868 w876 w911 w919 w994 w1011 w1090 w1109 w1124 w1129 w1136 w1151 w1158 w1262 w1333 w1340 w1346 w1357 w1364 w1371]
          tunnel: w89 -> [w458 w494 w512 w517 w526 w531 w537 w581 w659 w697 w718 w727 w746 w771 w798 w799 w810 w841 w842 w862 w869 w877 w909 w915 w997 w1014 w1091 w1110 w1125 w1132 w1141 w1152 w1168 w1270 w1334 w1341 w1347 w1358 w1365 w1369]
          tunnel: [w458 w495 w512 w516 w526 w531 w537 w581 w659 w698 w718 w726 w746 w771 w797 w799 w809 w841 w856 w862 w869 w877 w909 w914 w997 w1014 w1091 w1110 w1125 w1132 w1141 w1152 w1167 w1270 w1334 w1341 w1347 w1358 w1365 w1369] -> w90
          tunnel: "mode buttons" -> [_ _ _ _ _ _ _ _ _ _ w717 _ _ _ _ _ _ _ _ _ _ _ _ _ _ _ _ _ _ _ _ _ _ _ _ _ _ _ _ _]
          tunnel: [w455 w497 w511 w515 w523 w528 w535 w577 w658 w688 w715 w723 w745 w770 w795 w802 w807 w839 w848 w865 w868 w876 w911 w919 w996 w1013 w1090 w1109 w1124 w1128 w1136 w1151 w1163 w1261 w1333 w1340 w1346 w1357 w1364 w1371] -> w91
          tunnel: [_ _ _ _ TRUE _ _ _ _ _ _ _ _ _ _ _ _ _ _ _ _ _ _ _ _ _ w1078 _ _ _ _ _ _ _ _ _ _ _ _ _] -> w166
          tunnel: w124 -> [w452 w492 w510 w514 w521 w530 w534 w576 w657 w692 w714 w722 w741 w758 w785 w801 w804 w840 w843 w864 w867 w871 w910 w918 w993 w1012 w1085 w1108 w1114 w1131 w1140 w1150 w1176 w1269 w1329 w1336 w1343 w1356 w1360 w1368]
          tunnel: [w452 w492 w510 w514 w521 w530 w534 w576 w657 w692 w714 w722 w741 w758 w785 w801 w804 w840 w843 w864 w867 w871 w910 w918 w993 w1012 w1089 w1108 w1114 w1131 w1140 w1150 w1176 w1263 w1328 w1335 w1342 w1356 w1359 w1368] -> w123
          tunnel: w113 -> [_ _ _ _ _ _ _ _ _ _ _ _ _ _ _ _ _ _ _ _ _ _ _ _ _ _ _ _ _ _ w1139 _ _ w1265 _ _ _ _ _ _]
          tunnel: w112 -> [_ _ _ _ _ _ _ _ _ _ _ _ _ _ _ _ _ _ _ _ _ _ _ _ _ _ _ _ _ _ w1138 _ _ w1264 _ _ _ _ _ _]
          tunnel: w93 -> [_ _ _ _ _ _ _ _ _ _ _ _ _ _ _ _ _ _ _ _ _ _ _ _ _ _ _ _ _ _ _ _ _ w1267 _ _ _ w1350 _ _]
          tunnel: w92 -> [_ _ _ _ _ _ _ _ _ _ _ _ _ _ _ _ _ _ _ _ _ _ _ _ _ _ _ _ _ _ _ _ _ w1266 _ _ _ w1349 _ _]
          tunnel: w88 -> [_ _ _ _ _ _ _ _ _ _ _ _ _ _ _ _ _ _ _ _ _ _ _ w913 _ _ _ _ _ _ _ _ w1154 _ _ _ _ _ _ _]
          frame "(qsm) schedule" {
            # "action buttons"
            # "Schedule tasks -- Use a selector tree (illustrated below), case structures, or other logic to specify state sequences (\"tasks\") to be performed in response to front-panel action buttons and flags set or cleared in other states."
            n38 = Unbundle By Name(w455) -> ("State"=w454:T1)
            n39 = case shown="\"(auto) Go Back\"" w454 {
              tunnel: [w460 w461 w462 w464 w465 _ _ _ _ _ _ _ _ _ w466 w467 w468 w469 w470 w471 w472 w473 w474 w475 w476 w478 w479 w480 w482 w483 w484 w485] -> w453
              frame "Align", Default {
                w460 = T34 [enum."Setup get", enum."Setup manipulator", enum."(auto) Count balls", enum."(auto) Analyze balls", enum."(image) show"] items=["(qsm) schedule", "(qsm) initialize", "(qsm) release", "(qsm) clean up", "(qsm) shutdown", "(myRIO) initialize", "(myRIO) clean up", "(myRIO) update ports", "Setup get", "(image) get", "(image) show", "(ball) Shape detection", "(ball) Calc ball indx", "(ball) Calculate ROI", "(ball) Analyze color", "(ball) Align", "(ball) Wait", "(ball) Grab", "(pattern) Find Square", "(pattern) Calculate ROI", "(pattern) Calc pattern indx", "Compare", "(pattern) Analyze pattern", "(pattern) Align", "(pattern) Wait", "(pattern) states control", "navx", "stop motors", "(joystick) Joystick control", "_Timer", "Setup manipulator", "(auto) Count balls", "(auto) Analyze balls", "(auto) Dot Controller", "(auto) Fwd (cm)", "(auto) Turn (angle)", "(auto) Tnl (M2-M2.5)", "(auto) Recover Def Pos", "(auto) Go Back Controller", "Wait for button"]
                n40 = local write "Manip state"(enum16{"Align", "Grab", "Release"}."Align" ("Manip state")) -> ()
              }
              frame "1" {
                w461 = T34 [enum."Setup get", enum."(pattern) Align", enum."(auto) Fwd (cm)", enum."(myRIO) update ports", enum."(auto) Dot Controller"] items=["(qsm) schedule", "(qsm) initialize", "(qsm) release", "(qsm) clean up", "(qsm) shutdown", "(myRIO) initialize", "(myRIO) clean up", "(myRIO) update ports", "Setup get", "(image) get", "(image) show", "(ball) Shape detection", "(ball) Calc ball indx", "(ball) Calculate ROI", "(ball) Analyze color", "(ball) Align", "(ball) Wait", "(ball) Grab", "(pattern) Find Square", "(pattern) Calculate ROI", "(pattern) Calc pattern indx", "Compare", "(pattern) Analyze pattern", "(pattern) Align", "(pattern) Wait", "(pattern) states control", "navx", "stop motors", "(joystick) Joystick control", "_Timer", "Setup manipulator", "(auto) Count balls", "(auto) Analyze balls", "(auto) Dot Controller", "(auto) Fwd (cm)", "(auto) Turn (angle)", "(auto) Tnl (M2-M2.5)", "(auto) Recover Def Pos", "(auto) Go Back Controller", "Wait for button"]
              }
              frame "2" {
                w462 = T34 [enum."Setup get", enum."(pattern) Align", enum."(auto) Turn (angle)", enum."(myRIO) update ports", enum."(auto) Dot Controller"] items=["(qsm) schedule", "(qsm) initialize", "(qsm) release", "(qsm) clean up", "(qsm) shutdown", "(myRIO) initialize", "(myRIO) clean up", "(myRIO) update ports", "Setup get", "(image) get", "(image) show", "(ball) Shape detection", "(ball) Calc ball indx", "(ball) Calculate ROI", "(ball) Analyze color", "(ball) Align", "(ball) Wait", "(ball) Grab", "(pattern) Find Square", "(pattern) Calculate ROI", "(pattern) Calc pattern indx", "Compare", "(pattern) Analyze pattern", "(pattern) Align", "(pattern) Wait", "(pattern) states control", "navx", "stop motors", "(joystick) Joystick control", "_Timer", "Setup manipulator", "(auto) Count balls", "(auto) Analyze balls", "(auto) Dot Controller", "(auto) Fwd (cm)", "(auto) Turn (angle)", "(auto) Tnl (M2-M2.5)", "(auto) Recover Def Pos", "(auto) Go Back Controller", "Wait for button"]
              }
              frame "3" {
                w464 = T34 [enum."Setup get", enum."Setup manipulator", enum."(auto) Tnl (M2-M2.5)", enum."(myRIO) update ports", enum."(auto) Dot Controller"] items=["(qsm) schedule", "(qsm) initialize", "(qsm) release", "(qsm) clean up", "(qsm) shutdown", "(myRIO) initialize", "(myRIO) clean up", "(myRIO) update ports", "Setup get", "(image) get", "(image) show", "(ball) Shape detection", "(ball) Calc ball indx", "(ball) Calculate ROI", "(ball) Analyze color", "(ball) Align", "(ball) Wait", "(ball) Grab", "(pattern) Find Square", "(pattern) Calculate ROI", "(pattern) Calc pattern indx", "Compare", "(pattern) Analyze pattern", "(pattern) Align", "(pattern) Wait", "(pattern) states control", "navx", "stop motors", "(joystick) Joystick control", "_Timer", "Setup manipulator", "(auto) Count balls", "(auto) Analyze balls", "(auto) Dot Controller", "(auto) Fwd (cm)", "(auto) Turn (angle)", "(auto) Tnl (M2-M2.5)", "(auto) Recover Def Pos", "(auto) Go Back Controller", "Wait for button"]
                n41 = local write "Manip state"(enum16{"Align", "Grab", "Release"}."Release" ("Manip state")) -> ()
              }
              frame "4" {
                w465 = T34 [enum."_Timer"] items=["(qsm) schedule", "(qsm) initialize", "(qsm) release", "(qsm) clean up", "(qsm) shutdown", "(myRIO) initialize", "(myRIO) clean up", "(myRIO) update ports", "Setup get", "(image) get", "(image) show", "(ball) Shape detection", "(ball) Calc ball indx", "(ball) Calculate ROI", "(ball) Analyze color", "(ball) Align", "(ball) Wait", "(ball) Grab", "(pattern) Find Square", "(pattern) Calculate ROI", "(pattern) Calc pattern indx", "Compare", "(pattern) Analyze pattern", "(pattern) Align", "(pattern) Wait", "(pattern) states control", "navx", "stop motors", "(joystick) Joystick control", "_Timer", "Setup manipulator", "(auto) Count balls", "(auto) Analyze balls", "(auto) Dot Controller", "(auto) Fwd (cm)", "(auto) Turn (angle)", "(auto) Tnl (M2-M2.5)", "(auto) Recover Def Pos", "(auto) Go Back Controller", "Wait for button"]
              }
              frame "5" {
              }
              frame "6" {
              }
              frame "7" {
              }
              frame "8" {
              }
              frame "9" {
              }
              frame "10" {
              }
              frame "11" {
              }
              frame "12" {
              }
              frame "13" {
              }
              frame "(pattern) Align" {
                w466 = T34 [enum."Setup get", enum."(image) get", enum."(pattern) Find Square", enum."(pattern) Align", enum."(pattern) Wait", enum."(myRIO) update ports"] items=["(qsm) schedule", "(qsm) initialize", "(qsm) release", "(qsm) clean up", "(qsm) shutdown", "(myRIO) initialize", "(myRIO) clean up", "(myRIO) update ports", "Setup get", "(image) get", "(image) show", "(ball) Shape detection", "(ball) Calc ball indx", "(ball) Calculate ROI", "(ball) Analyze color", "(ball) Align", "(ball) Wait", "(ball) Grab", "(pattern) Find Square", "(pattern) Calculate ROI", "(pattern) Calc pattern indx", "Compare", "(pattern) Analyze pattern", "(pattern) Align", "(pattern) Wait", "(pattern) states control", "navx", "stop motors", "(joystick) Joystick control", "_Timer", "Setup manipulator", "(auto) Count balls", "(auto) Analyze balls", "(auto) Dot Controller", "(auto) Fwd (cm)", "(auto) Turn (angle)", "(auto) Tnl (M2-M2.5)", "(auto) Recover Def Pos", "(auto) Go Back Controller", "Wait for button"] ("task")
              }
              frame "Pattern" {
                w467 = T34 [enum."Setup get", enum."(image) get", enum."(pattern) Find Square", enum."(pattern) Calculate ROI", enum."(pattern) Calc pattern indx", enum."(pattern) Analyze pattern", enum."(image) show", enum."(myRIO) update ports", enum."Wait for button"] items=["(qsm) schedule", "(qsm) initialize", "(qsm) release", "(qsm) clean up", "(qsm) shutdown", "(myRIO) initialize", "(myRIO) clean up", "(myRIO) update ports", "Setup get", "(image) get", "(image) show", "(ball) Shape detection", "(ball) Calc ball indx", "(ball) Calculate ROI", "(ball) Analyze color", "(ball) Align", "(ball) Wait", "(ball) Grab", "(pattern) Find Square", "(pattern) Calculate ROI", "(pattern) Calc pattern indx", "Compare", "(pattern) Analyze pattern", "(pattern) Align", "(pattern) Wait", "(pattern) states control", "navx", "stop motors", "(joystick) Joystick control", "_Timer", "Setup manipulator", "(auto) Count balls", "(auto) Analyze balls", "(auto) Dot Controller", "(auto) Fwd (cm)", "(auto) Turn (angle)", "(auto) Tnl (M2-M2.5)", "(auto) Recover Def Pos", "(auto) Go Back Controller", "Wait for button"] ("task")
              }
              frame "(mod) pattern" {
                w468 = T34 [enum."Setup get", enum."_Timer", enum."(image) get", enum."(pattern) Find Square", enum."(pattern) Calculate ROI", enum."(pattern) Analyze pattern", enum."Compare", enum."(pattern) Calc pattern indx", enum."(image) show", enum."(myRIO) update ports", enum."Wait for button"] items=["(qsm) schedule", "(qsm) initialize", "(qsm) release", "(qsm) clean up", "(qsm) shutdown", "(myRIO) initialize", "(myRIO) clean up", "(myRIO) update ports", "Setup get", "(image) get", "(image) show", "(ball) Shape detection", "(ball) Calc ball indx", "(ball) Calculate ROI", "(ball) Analyze color", "(ball) Align", "(ball) Wait", "(ball) Grab", "(pattern) Find Square", "(pattern) Calculate ROI", "(pattern) Calc pattern indx", "Compare", "(pattern) Analyze pattern", "(pattern) Align", "(pattern) Wait", "(pattern) states control", "navx", "stop motors", "(joystick) Joystick control", "_Timer", "Setup manipulator", "(auto) Count balls", "(auto) Analyze balls", "(auto) Dot Controller", "(auto) Fwd (cm)", "(auto) Turn (angle)", "(auto) Tnl (M2-M2.5)", "(auto) Recover Def Pos", "(auto) Go Back Controller", "Wait for button"] ("task")
              }
              frame "<mod>[P] remembering" {
                w469 = T34 [enum."Setup get", enum."_Timer", enum."(image) get", enum."(pattern) Find Square", enum."(pattern) Calculate ROI", enum."(pattern) Analyze pattern", enum."(pattern) Calc pattern indx", enum."(image) show", enum."(myRIO) update ports", enum."Wait for button", enum."(pattern) states control"] items=["(qsm) schedule", "(qsm) initialize", "(qsm) release", "(qsm) clean up", "(qsm) shutdown", "(myRIO) initialize", "(myRIO) clean up", "(myRIO) update ports", "Setup get", "(image) get", "(image) show", "(ball) Shape detection", "(ball) Calc ball indx", "(ball) Calculate ROI", "(ball) Analyze color", "(ball) Align", "(ball) Wait", "(ball) Grab", "(pattern) Find Square", "(pattern) Calculate ROI", "(pattern) Calc pattern indx", "Compare", "(pattern) Analyze pattern", "(pattern) Align", "(pattern) Wait", "(pattern) states control", "navx", "stop motors", "(joystick) Joystick control", "_Timer", "Setup manipulator", "(auto) Count balls", "(auto) Analyze balls", "(auto) Dot Controller", "(auto) Fwd (cm)", "(auto) Turn (angle)", "(auto) Tnl (M2-M2.5)", "(auto) Recover Def Pos", "(auto) Go Back Controller", "Wait for button"] ("task")
              }
              frame "<mod>[P] go through tunnel" {
                w470 = T34 [enum."Setup get", enum."_Timer", enum."(image) get", enum."(pattern) Find Square", enum."(pattern) Calculate ROI", enum."(pattern) Analyze pattern", enum."(pattern) Calc pattern indx", enum."(image) show", enum."(myRIO) update ports", enum."Wait for button", enum."(pattern) states control"] items=["(qsm) schedule", "(qsm) initialize", "(qsm) release", "(qsm) clean up", "(qsm) shutdown", "(myRIO) initialize", "(myRIO) clean up", "(myRIO) update ports", "Setup get", "(image) get", "(image) show", "(ball) Shape detection", "(ball) Calc ball indx", "(ball) Calculate ROI", "(ball) Analyze color", "(ball) Align", "(ball) Wait", "(ball) Grab", "(pattern) Find Square", "(pattern) Calculate ROI", "(pattern) Calc pattern indx", "Compare", "(pattern) Analyze pattern", "(pattern) Align", "(pattern) Wait", "(pattern) states control", "navx", "stop motors", "(joystick) Joystick control", "_Timer", "Setup manipulator", "(auto) Count balls", "(auto) Analyze balls", "(auto) Dot Controller", "(auto) Fwd (cm)", "(auto) Turn (angle)", "(auto) Tnl (M2-M2.5)", "(auto) Recover Def Pos", "(auto) Go Back Controller", "Wait for button"] ("task")
              }
              frame "<mod>[P] comparing" {
                w471 = T34 [enum."Setup get", enum."_Timer", enum."(image) get", enum."(pattern) Find Square", enum."(qsm) schedule", enum."(pattern) Calculate ROI", enum."(pattern) Analyze pattern", enum."(pattern) Calc pattern indx", enum."(image) show", enum."(myRIO) update ports", enum."Wait for button", enum."(pattern) states control"] items=["(qsm) schedule", "(qsm) initialize", "(qsm) release", "(qsm) clean up", "(qsm) shutdown", "(myRIO) initialize", "(myRIO) clean up", "(myRIO) update ports", "Setup get", "(image) get", "(image) show", "(ball) Shape detection", "(ball) Calc ball indx", "(ball) Calculate ROI", "(ball) Analyze color", "(ball) Align", "(ball) Wait", "(ball) Grab", "(pattern) Find Square", "(pattern) Calculate ROI", "(pattern) Calc pattern indx", "Compare", "(pattern) Analyze pattern", "(pattern) Align", "(pattern) Wait", "(pattern) states control", "navx", "stop motors", "(joystick) Joystick control", "_Timer", "Setup manipulator", "(auto) Count balls", "(auto) Analyze balls", "(auto) Dot Controller", "(auto) Fwd (cm)", "(auto) Turn (angle)", "(auto) Tnl (M2-M2.5)", "(auto) Recover Def Pos", "(auto) Go Back Controller", "Wait for button"] ("task")
              }
              frame "(mod) ball" {
                w472 = T34 [enum."(image) get", enum."(image) get", enum."(ball) Shape detection", enum."(ball) Calculate ROI", enum."(ball) Analyze color", enum."Compare", enum."(ball) Calc ball indx", enum."(image) show", enum."(myRIO) update ports", enum."Wait for button"] items=["(qsm) schedule", "(qsm) initialize", "(qsm) release", "(qsm) clean up", "(qsm) shutdown", "(myRIO) initialize", "(myRIO) clean up", "(myRIO) update ports", "Setup get", "(image) get", "(image) show", "(ball) Shape detection", "(ball) Calc ball indx", "(ball) Calculate ROI", "(ball) Analyze color", "(ball) Align", "(ball) Wait", "(ball) Grab", "(pattern) Find Square", "(pattern) Calculate ROI", "(pattern) Calc pattern indx", "Compare", "(pattern) Analyze pattern", "(pattern) Align", "(pattern) Wait", "(pattern) states control", "navx", "stop motors", "(joystick) Joystick control", "_Timer", "Setup manipulator", "(auto) Count balls", "(auto) Analyze balls", "(auto) Dot Controller", "(auto) Fwd (cm)", "(auto) Turn (angle)", "(auto) Tnl (M2-M2.5)", "(auto) Recover Def Pos", "(auto) Go Back Controller", "Wait for button"] ("task")
              }
              frame "Ball" {
                w473 = T34 [enum."(image) get", enum."(ball) Shape detection", enum."(ball) Calculate ROI", enum."(ball) Calc ball indx", enum."(ball) Analyze color", enum."(image) show", enum."Wait for button", enum."(myRIO) update ports"] items=["(qsm) schedule", "(qsm) initialize", "(qsm) release", "(qsm) clean up", "(qsm) shutdown", "(myRIO) initialize", "(myRIO) clean up", "(myRIO) update ports", "Setup get", "(image) get", "(image) show", "(ball) Shape detection", "(ball) Calc ball indx", "(ball) Calculate ROI", "(ball) Analyze color", "(ball) Align", "(ball) Wait", "(ball) Grab", "(pattern) Find Square", "(pattern) Calculate ROI", "(pattern) Calc pattern indx", "Compare", "(pattern) Analyze pattern", "(pattern) Align", "(pattern) Wait", "(pattern) states control", "navx", "stop motors", "(joystick) Joystick control", "_Timer", "Setup manipulator", "(auto) Count balls", "(auto) Analyze balls", "(auto) Dot Controller", "(auto) Fwd (cm)", "(auto) Turn (angle)", "(auto) Tnl (M2-M2.5)", "(auto) Recover Def Pos", "(auto) Go Back Controller", "Wait for button"] ("task")
              }
              frame "Other" {
                w474 = T34 [enum."(image) get", enum."(pattern) Find Square", enum."(pattern) Calculate ROI", enum."(pattern) Analyze pattern", enum."(image) show", enum."Wait for button", enum."(myRIO) update ports", enum."(image) get", enum."(ball) Shape detection", enum."(ball) Calculate ROI", enum."(ball) Analyze color", enum."(image) show", enum."Wait for button", enum."(myRIO) update ports"] items=["(qsm) schedule", "(qsm) initialize", "(qsm) release", "(qsm) clean up", "(qsm) shutdown", "(myRIO) initialize", "(myRIO) clean up", "(myRIO) update ports", "Setup get", "(image) get", "(image) show", "(ball) Shape detection", "(ball) Calc ball indx", "(ball) Calculate ROI", "(ball) Analyze color", "(ball) Align", "(ball) Wait", "(ball) Grab", "(pattern) Find Square", "(pattern) Calculate ROI", "(pattern) Calc pattern indx", "Compare", "(pattern) Analyze pattern", "(pattern) Align", "(pattern) Wait", "(pattern) states control", "navx", "stop motors", "(joystick) Joystick control", "_Timer", "Setup manipulator", "(auto) Count balls", "(auto) Analyze balls", "(auto) Dot Controller", "(auto) Fwd (cm)", "(auto) Turn (angle)", "(auto) Tnl (M2-M2.5)", "(auto) Recover Def Pos", "(auto) Go Back Controller", "Wait for button"] ("task")
              }
              frame "Clear" {
                w475 = T34 [enum."Setup get", enum."(ball) Grab", enum."(auto) Dot Controller"] items=["(qsm) schedule", "(qsm) initialize", "(qsm) release", "(qsm) clean up", "(qsm) shutdown", "(myRIO) initialize", "(myRIO) clean up", "(myRIO) update ports", "Setup get", "(image) get", "(image) show", "(ball) Shape detection", "(ball) Calc ball indx", "(ball) Calculate ROI", "(ball) Analyze color", "(ball) Align", "(ball) Wait", "(ball) Grab", "(pattern) Find Square", "(pattern) Calculate ROI", "(pattern) Calc pattern indx", "Compare", "(pattern) Analyze pattern", "(pattern) Align", "(pattern) Wait", "(pattern) states control", "navx", "stop motors", "(joystick) Joystick control", "_Timer", "Setup manipulator", "(auto) Count balls", "(auto) Analyze balls", "(auto) Dot Controller", "(auto) Fwd (cm)", "(auto) Turn (angle)", "(auto) Tnl (M2-M2.5)", "(auto) Recover Def Pos", "(auto) Go Back Controller", "Wait for button"] ("task")
              }
              frame "navx" {
                w476 = T34 [enum."(auto) Dot Controller"] items=["(qsm) schedule", "(qsm) initialize", "(qsm) release", "(qsm) clean up", "(qsm) shutdown", "(myRIO) initialize", "(myRIO) clean up", "(myRIO) update ports", "Setup get", "(image) get", "(image) show", "(ball) Shape detection", "(ball) Calc ball indx", "(ball) Calculate ROI", "(ball) Analyze color", "(ball) Align", "(ball) Wait", "(ball) Grab", "(pattern) Find Square", "(pattern) Calculate ROI", "(pattern) Calc pattern indx", "Compare", "(pattern) Analyze pattern", "(pattern) Align", "(pattern) Wait", "(pattern) states control", "navx", "stop motors", "(joystick) Joystick control", "_Timer", "Setup manipulator", "(auto) Count balls", "(auto) Analyze balls", "(auto) Dot Controller", "(auto) Fwd (cm)", "(auto) Turn (angle)", "(auto) Tnl (M2-M2.5)", "(auto) Recover Def Pos", "(auto) Go Back Controller", "Wait for button"]
              }
              frame "(auto) Balls Analyze" {
                w478 = T34 [enum."Setup get", enum."Setup manipulator", enum."(image) get", enum."(ball) Shape detection", enum."(auto) Count balls", enum."(auto) Analyze balls", enum."(myRIO) update ports"] items=["(qsm) schedule", "(qsm) initialize", "(qsm) release", "(qsm) clean up", "(qsm) shutdown", "(myRIO) initialize", "(myRIO) clean up", "(myRIO) update ports", "Setup get", "(image) get", "(image) show", "(ball) Shape detection", "(ball) Calc ball indx", "(ball) Calculate ROI", "(ball) Analyze color", "(ball) Align", "(ball) Wait", "(ball) Grab", "(pattern) Find Square", "(pattern) Calculate ROI", "(pattern) Calc pattern indx", "Compare", "(pattern) Analyze pattern", "(pattern) Align", "(pattern) Wait", "(pattern) states control", "navx", "stop motors", "(joystick) Joystick control", "_Timer", "Setup manipulator", "(auto) Count balls", "(auto) Analyze balls", "(auto) Dot Controller", "(auto) Fwd (cm)", "(auto) Turn (angle)", "(auto) Tnl (M2-M2.5)", "(auto) Recover Def Pos", "(auto) Go Back Controller", "Wait for button"] ("task")
                n42 = local write "Manip state"(enum16{"Align", "Grab", "Release"}."Align" ("Manip state")) -> ()
              }
              frame "(auto) Ball Analyze" {
                w479 = T34 [enum."(ball) Calculate ROI", enum."(ball) Analyze color", enum."(auto) Analyze balls"] items=["(qsm) schedule", "(qsm) initialize", "(qsm) release", "(qsm) clean up", "(qsm) shutdown", "(myRIO) initialize", "(myRIO) clean up", "(myRIO) update ports", "Setup get", "(image) get", "(image) show", "(ball) Shape detection", "(ball) Calc ball indx", "(ball) Calculate ROI", "(ball) Analyze color", "(ball) Align", "(ball) Wait", "(ball) Grab", "(pattern) Find Square", "(pattern) Calculate ROI", "(pattern) Calc pattern indx", "Compare", "(pattern) Analyze pattern", "(pattern) Align", "(pattern) Wait", "(pattern) states control", "navx", "stop motors", "(joystick) Joystick control", "_Timer", "Setup manipulator", "(auto) Count balls", "(auto) Analyze balls", "(auto) Dot Controller", "(auto) Fwd (cm)", "(auto) Turn (angle)", "(auto) Tnl (M2-M2.5)", "(auto) Recover Def Pos", "(auto) Go Back Controller", "Wait for button"] ("task")
              }
              frame "(pattern) Align <loop>" {
                w480 = T34 [enum."Setup get", enum."(image) get", enum."(pattern) Find Square", enum."(pattern) Align", enum."(pattern) Wait", enum."(myRIO) update ports"] items=["(qsm) schedule", "(qsm) initialize", "(qsm) release", "(qsm) clean up", "(qsm) shutdown", "(myRIO) initialize", "(myRIO) clean up", "(myRIO) update ports", "Setup get", "(image) get", "(image) show", "(ball) Shape detection", "(ball) Calc ball indx", "(ball) Calculate ROI", "(ball) Analyze color", "(ball) Align", "(ball) Wait", "(ball) Grab", "(pattern) Find Square", "(pattern) Calculate ROI", "(pattern) Calc pattern indx", "Compare", "(pattern) Analyze pattern", "(pattern) Align", "(pattern) Wait", "(pattern) states control", "navx", "stop motors", "(joystick) Joystick control", "_Timer", "Setup manipulator", "(auto) Count balls", "(auto) Analyze balls", "(auto) Dot Controller", "(auto) Fwd (cm)", "(auto) Turn (angle)", "(auto) Tnl (M2-M2.5)", "(auto) Recover Def Pos", "(auto) Go Back Controller", "Wait for button"] ("task")
              }
              frame "(ball) Align <loop>" {
                w482 = T34 [enum."Setup get", enum."Setup manipulator", enum."(image) get", enum."(ball) Shape detection", enum."(ball) Align", enum."(ball) Wait", enum."(auto) Count balls", enum."(auto) Analyze balls", enum."(myRIO) update ports"] items=["(qsm) schedule", "(qsm) initialize", "(qsm) release", "(qsm) clean up", "(qsm) shutdown", "(myRIO) initialize", "(myRIO) clean up", "(myRIO) update ports", "Setup get", "(image) get", "(image) show", "(ball) Shape detection", "(ball) Calc ball indx", "(ball) Calculate ROI", "(ball) Analyze color", "(ball) Align", "(ball) Wait", "(ball) Grab", "(pattern) Find Square", "(pattern) Calculate ROI", "(pattern) Calc pattern indx", "Compare", "(pattern) Analyze pattern", "(pattern) Align", "(pattern) Wait", "(pattern) states control", "navx", "stop motors", "(joystick) Joystick control", "_Timer", "Setup manipulator", "(auto) Count balls", "(auto) Analyze balls", "(auto) Dot Controller", "(auto) Fwd (cm)", "(auto) Turn (angle)", "(auto) Tnl (M2-M2.5)", "(auto) Recover Def Pos", "(auto) Go Back Controller", "Wait for button"]
                n43 = local write "Manip state"(enum16{"Align", "Grab", "Release"}."Align" ("Manip state")) -> ()
              }
              frame "(auto) Recover Def Pos" {
                w483 = T34 [enum."(auto) Recover Def Pos", enum."(auto) Dot Controller"] items=["(qsm) schedule", "(qsm) initialize", "(qsm) release", "(qsm) clean up", "(qsm) shutdown", "(myRIO) initialize", "(myRIO) clean up", "(myRIO) update ports", "Setup get", "(image) get", "(image) show", "(ball) Shape detection", "(ball) Calc ball indx", "(ball) Calculate ROI", "(ball) Analyze color", "(ball) Align", "(ball) Wait", "(ball) Grab", "(pattern) Find Square", "(pattern) Calculate ROI", "(pattern) Calc pattern indx", "Compare", "(pattern) Analyze pattern", "(pattern) Align", "(pattern) Wait", "(pattern) states control", "navx", "stop motors", "(joystick) Joystick control", "_Timer", "Setup manipulator", "(auto) Count balls", "(auto) Analyze balls", "(auto) Dot Controller", "(auto) Fwd (cm)", "(auto) Turn (angle)", "(auto) Tnl (M2-M2.5)", "(auto) Recover Def Pos", "(auto) Go Back Controller", "Wait for button"]
              }
              frame "(auto) Go Back" {
                w484 = T34 [enum."(auto) Go Back Controller", enum."(qsm) shutdown"] items=["(qsm) schedule", "(qsm) initialize", "(qsm) release", "(qsm) clean up", "(qsm) shutdown", "(myRIO) initialize", "(myRIO) clean up", "(myRIO) update ports", "Setup get", "(image) get", "(image) show", "(ball) Shape detection", "(ball) Calc ball indx", "(ball) Calculate ROI", "(ball) Analyze color", "(ball) Align", "(ball) Wait", "(ball) Grab", "(pattern) Find Square", "(pattern) Calculate ROI", "(pattern) Calc pattern indx", "Compare", "(pattern) Analyze pattern", "(pattern) Align", "(pattern) Wait", "(pattern) states control", "navx", "stop motors", "(joystick) Joystick control", "_Timer", "Setup manipulator", "(auto) Count balls", "(auto) Analyze balls", "(auto) Dot Controller", "(auto) Fwd (cm)", "(auto) Turn (angle)", "(auto) Tnl (M2-M2.5)", "(auto) Recover Def Pos", "(auto) Go Back Controller", "Wait for button"]
              }
              frame "Joystick control" {
                w485 = T34 [enum."(joystick) Joystick control", enum."(myRIO) update ports"] items=["(qsm) schedule", "(qsm) initialize", "(qsm) release", "(qsm) clean up", "(qsm) shutdown", "(myRIO) initialize", "(myRIO) clean up", "(myRIO) update ports", "Setup get", "(image) get", "(image) show", "(ball) Shape detection", "(ball) Calc ball indx", "(ball) Calculate ROI", "(ball) Analyze color", "(ball) Align", "(ball) Wait", "(ball) Grab", "(pattern) Find Square", "(pattern) Calculate ROI", "(pattern) Calc pattern indx", "Compare", "(pattern) Analyze pattern", "(pattern) Align", "(pattern) Wait", "(pattern) states control", "navx", "stop motors", "(joystick) Joystick control", "_Timer", "Setup manipulator", "(auto) Count balls", "(auto) Analyze balls", "(auto) Dot Controller", "(auto) Fwd (cm)", "(auto) Turn (angle)", "(auto) Tnl (M2-M2.5)", "(auto) Recover Def Pos", "(auto) Go Back Controller", "Wait for button"]
              }
            }
            n44 = call "enqueue_states.vi"("task"=w453, "error in"=w456, "queue in"=w457) -> ("error out"=w451:errorcluster)  [unwired: 6 in, 1 out]
          }
          frame "(qsm) initialize" {
            w500 = T35 0 items=["Grayscale (U8)", "Grayscale (I16)", "Grayscale (SGL)", "Complex (CSG)", "RGB (U32)", "HSL (U32)", "RGB (U64)", "Grayscale (U16)"] ("Image Type")
            # "Initialize -- Allocate memory for additional image buffers, if necessary, and perform other one-time initialization steps."
            n45 = flat-sequence {
              frame #0 {
                n46 = Initialize Array(0 ("element"), "Dots in total") -> (→"Angles" →"Left_enc" →"Right_enc" →"M_enc" →"G_enc":i32[])
                n47 = local read "States in total"() -> (w505:i32)
                n48 = Initialize Array(0 ("element"), w505) -> (→"FT_Angles" →"FT_Left_enc" →"FT_Right_enc" →"FT_M_enc" →"FT_G_enc":i32[])
              }
            }
            n49 = Initialize Array(30, 16) -> (w487:i32[])
            n50 = call "IMAQ Create"("Border Size"=3, "Image Name"="img0", "Image Type"=w500, "error in (no error)"=w502) -> ("New Image"=w498:T8, "error out"=w486:errorcluster)  [unwired: 1 in]
            n51 = Initialize Array(20, 16) -> (w490:i32[])
            n52 = Bundle By Name(cluster=w494, "image ref"=w498) -> (w496:T11)
            n53 = Bundle By Name(cluster=w496, "Color classes"=w490, "Pattern classes"=w487) -> (w495:T11)
          }
          frame "(qsm) release" {
            # "Release all front-panel action buttons."
          }
          frame "(qsm) clean up" {
            # "Set the \"Stop webcam\" flag"
            # "Clean up -- Set the \"Stop webcam flag\" and perform other necessary clean-up actions."
            n54 = Bundle By Name(cluster=w517, "qsm.Stop webcam"=TRUE) -> (w516:T11)
          }
          frame "(qsm) shutdown" {
            # "deallocate image buffer memory"
            # "stop the loop"
            # "Shutdown -- Release the state queue, free all image buffer memory, and stop the while-loop structure."
            n55 = Release Queue(queue=w527, error in (no error)=w520) -> (error out=w524:errorcluster)  [unwired: 1 in, 2 out]
            n56 = call "Imaq Dispose"("All Images? (No)"=TRUE, "error in (no error)"=w524) -> ("error out"=w519:errorcluster)  [unwired: 4 in]
          }
          frame "(myRIO) initialize" {
            # "Initialize (myRIO) -- Open channels, configure devices, send setup strings to peripherals, etc."
          }
          frame "(myRIO) clean up" {
            w536 = FALSE ("LED3")
            # "clear the onboard LEDs"
            # "Clean up (myRIO) -- Return myRIO devices and external peripherals to inactive states."
            n57 = xnode "LED 3"("LED0"=w536, "LED1"=w536, "LED2"=w536, "LED3"=w536, "error in (no error)"=w533) -> ("error out"=w532:errorcluster)
          }
          frame "(myRIO) update ports" {
            # "show the button state\non the onboard LEDs"
            # "set the flag"
            # "press the onboard button\nto set the \"save image\" flag"
            # "Update ports (myRIO) -- Read and write onboard devices and external peripherals."
            n58 = xnode "Button"("error in (no error)"=w580) -> ("Value"=w578:bool, "error out"=w579:errorcluster)
            n59 = xnode "LED"("LED0"=w578, "LED1"=w578, "LED2"=w578, "LED3"=w578, "error in (no error)"=w579) -> ()  [unwired: 1 out]
          }
          frame "Setup get" {
            n60 = Unbundle By Name(w658) -> ("State"=w656:T1)
            n61 = flat-sequence {
              tunnel: w656 -> [w660]
              frame #0 {
                n62 = case shown="\"1\"" w660 {
                  frame "Align", Default {
                    n63 = local write "Camera state"(enum16{"Fwd", "Pattern", "Ball"}."Ball" ("Camera state")) -> ()
                    "rotate" <- FALSE ("rotate")
                  }
                  frame "1" {
                    n64 = local write "Camera state"(enum16{"Fwd", "Pattern", "Ball"}."Pattern" ("Camera state")) -> ()
                  }
                  frame "2" {
                  }
                  frame "3" {
                    n65 = local write "Camera state"(enum16{"Fwd", "Pattern", "Ball"}."Ball" ("Camera state")) -> ()
                  }
                  frame "4" {
                    n66 = local write "Camera state"(enum16{"Fwd", "Pattern", "Ball"}."Ball" ("Camera state")) -> ()
                  }
                  frame "5" {
                  }
                  frame "6" {
                  }
                  frame "7" {
                  }
                  frame "8" {
                  }
                  frame "9" {
                  }
                  frame "10" {
                  }
                  frame "11" {
                  }
                  frame "12" {
                  }
                  frame "13" {
                  }
                  frame "(pattern) Align" {
                    n67 = local write "rotate"(TRUE ("rotate")) -> ()
                    n68 = local write "Camera state"(enum16{"Fwd", "Pattern", "Ball"}."Pattern" ("Camera state")) -> ()
                  }
                  frame "Pattern" {
                    n69 = local write "Camera state"(enum16{"Fwd", "Pattern", "Ball"}."Pattern" ("Camera state")) -> ()
                  }
                  frame "(mod) pattern" {
                    n70 = local write "Camera state"(enum16{"Fwd", "Pattern", "Ball"}."Pattern" ("Camera state")) -> ()
                  }
                  frame "<mod>[P] remembering" {
                    n71 = local write "Camera state"(enum16{"Fwd", "Pattern", "Ball"}."Pattern" ("Camera state")) -> ()
                  }
                  frame "<mod>[P] go through tunnel" {
                    n72 = local write "Camera state"(enum16{"Fwd", "Pattern", "Ball"}."Pattern" ("Camera state")) -> ()
                  }
                  frame "<mod>[P] comparing" {
                    n73 = local write "Camera state"(enum16{"Fwd", "Pattern", "Ball"}."Pattern" ("Camera state")) -> ()
                  }
                  frame "(mod) ball" {
                    n74 = local write "Camera state"(enum16{"Fwd", "Pattern", "Ball"}."Ball" ("Camera state")) -> ()
                  }
                  frame "Ball" {
                    n75 = local write "Camera state"(enum16{"Fwd", "Pattern", "Ball"}."Ball" ("Camera state")) -> ()
                  }
                  frame "Other" {
                  }
                  frame "Clear" {
                    n76 = local write "Camera state"(enum16{"Fwd", "Pattern", "Ball"}."Ball" ("Camera state")) -> ()
                  }
                  frame "navx" {
                  }
                  frame "(auto) Balls Analyze" {
                    n77 = local write "Camera state"(enum16{"Fwd", "Pattern", "Ball"}."Ball" ("Camera state")) -> ()
                    n78 = local write "rotate"(FALSE ("rotate")) -> ()
                  }
                  frame "(auto) Ball Analyze" {
                  }
                  frame "(pattern) Align <loop>" {
                  }
                  frame "(ball) Align <loop>" {
                  }
                  frame "Joystick control" {
                  }
                }
              }
              frame #1 {
                n79 = call "Setup camera (SubVI).vi"("M duty cycle [P]"="M duty cycle [P]", "S duty cycle [B]   in"="S duty cycle [B]", "M duty cycle [B]  in"="M duty cycle [B]", "S duty cycle [F]"="S duty cycle [F]", "M duty cycle [F]"="M duty cycle [F]", "Camera state"="Camera state", "S duty cycle [P]"="S duty cycle [P]") -> ("M duty cycle [B]  out"=w679:dbl, "S duty cycle [B]   out"=w680:dbl)  [unwired: 3 in]
                n80 = local write "[cur] duty cycle [%] (s)"(w680) -> ()
                n81 = local write "[cur] duty cycle [%] (m)"(w679) -> ()
              }
            }
          }
          frame "(image) get" {
            # "NOTE:\n1. Use NI-MAX to configure your webcam with the\n     *same* resolution (\"mode\") and attributes as those used \n     to develop your Vision Assistant script, especially if the\n     script depends on absolute ROIs, calibration images, template\n     images, background levels, etc.\n \n     Click \"Save\" to create or update the camera configuration files\n     on the target.\n\n2. Open the Vision Acquisition Express VI above and then\n     select \"Reset to Defaults\" to read the camera configuration\n     files created/updated by NI-MAX in the previous step."
            # "webcam image buffer is\ncreated during the first\ncall of the Vision\nAcquisition Express VI"
            # "Get image -- Retrieve a single webcam image frame and optionally flip the image right side up."
            n82 = call "Vision Acquisition"("error in"=w695) -> ("Image Out"=w693:T8, "error out"=w694:errorcluster)  [unwired: 24 in, 1 out]
            n83 = local read "rotate"() -> (w696:bool)
            n84 = case shown="True" w696 {
              tunnel: w693 -> [w707 w712]
              tunnel: [w707 w711] -> w691
              tunnel: w694 -> [w706 w709]
              tunnel: [w706 w710] -> w690
              frame False {
                # "use webcam image as-is"
              }
              frame True {
                # "rotate img for pattern"
                n85 = call "IMAQ Rotate"("error in (no error)"=w709, "Angle (degrees)"="Angle for pattern (degrees)", "Image Src"=w712) -> ("error out"=w710:errorcluster, "Image Dst Out"=w711:T8)  [unwired: 7 in]
              }
            }
            n86 = Unbundle By Name(w688) -> ("State"=w687:T1)
            n87 = case shown="\"Align\", Default" w687 {
              tunnel: w691 -> [w700 w705]
              tunnel: w690 -> [w699 w702]
              tunnel: [w700 w704] -> w689
              tunnel: [w699 w703] -> _
              frame "Align", Default {
              }
              frame "(pattern) Align" {
                n88 = call "IMAQ Rotate"("error in (no error)"=w702, "Angle (degrees)"="Angle for Align (degrees)", "Image Src"=w705) -> ("error out"=w703:errorcluster, "Image Dst Out"=w704:T8)  [unwired: 7 in]
              }
            }
            n89 = Bundle By Name(cluster=w697, "qsm.Webcam image ref"=w689) -> (w698:T11)
          }
          frame "(image) show" {
            # "Show image -- Select from among the available image buffers to show on the main image display; use a selector tree or case structure."
            n90 = Unbundle By Name "Unbundle By Name"(w717) -> ("show analyzed"=w716:bool)
            n91 = Unbundle By Name "Unbundle By Name"(w718) -> ("qsm.Analyzed image ref"=w721:T8, "qsm.Webcam image ref"=w720:T8)
            n92 = Select(t=w721, s=w716, f=w720) -> (s? t:f=→"image display":T8)
          }
          frame "(ball) Shape detection" {
            # "Shape detection"
            # "Expansion State A"
            n93 = Unbundle By Name(w727) -> ("qsm.Webcam image ref"=w729:T8)
            n94 = call "Vision Assistant"("Image In"=w729, "error in"=w730) -> ("Image Out"=w728:T8, "Circles Calibrated (Shape Detection 1)"=w724:T4, "Number of Matches (Shape Detection 1)"=→"Number of Matches (Shape Detection 1)":i32)  [unwired: 22 in, 1 out]
            "Circles Calibrated (Shape Detection 1)" <- w724
            n95 = disable-structure shown="Disabled" {
              disable-tunnel: w724 -> [w739 _]
              frame Disabled {
                n96 = Index Array(array=w739, index=0) -> (element=w737:T36)
                n97 = Unbundle By Name(w737) -> ("Position"=w736:cluster{"X":sgl, "Y":sgl}, "Radius"=→"CircleRadius":dbl)
                n98 = Unbundle(w736) -> ("X"=w735:sgl, "Y"=w734:sgl)
                n99 = To Double Precision Float(number=w735) -> (double precision float=→"curX":dbl)
                n100 = To Double Precision Float(number=w734) -> (double precision float=→"curY":dbl)
              }
              frame Enabled {
              }
            }
            n101 = Bundle By Name(cluster=w727, "qsm.Analyzed image ref"=w728) -> (w726:T11)
          }
          frame "(ball) Calc ball indx" {
            n102 = Unbundle By Name(w745) -> ("State"=w742:T1)
            n103 = Equal?(x=w742, y=T31."(mod) ball" ("Shape - t, Color - f")) -> (x = y?=w744:bool)
            n104 = case shown="True" w744 {
              frame False {
                n105 = local read "Circles Calibrated (Shape Detection 1)"() -> (w751:T4)
                n106 = control-ref of="Ball number"() -> (w753:refnum<vi>)
                n107 = control-ref of="Number of Matches (Shape Detection 1)"() -> (w754:refnum<vi>)
                n108 = local read "curX"() -> (w750:dbl)
                n109 = local read "curY"() -> (w749:dbl)
                n110 = To Single Precision Float(number=w750) -> (single precision float=w748:sgl)
                n111 = To Single Precision Float(number=w749) -> (single precision float=w747:sgl)
                n112 = call "Ball Index (SubVI).vi"("cur pos Y"=w747, "cur pos X"=w748, "Circles Calibrated (Shape Detection 1)"=w751, "Ball index"="Ball number", "reference in"=w753, "Digital in"=w754) -> ()  [unwired: 4 in]
              }
              frame True {
                n113 = local read "Ball number"() -> (w756:i32)
                n114 = Increment(x=w756) -> (x+1=w755:i32)
                n115 = local write "Ball number"(w755) -> ()
              }
            }
          }
          frame "(ball) Calculate ROI" {
            n116 = local read "Number of Matches (Shape Detection 1)"() -> (w768:i32)
            n117 = Greater Than 0?(x=w768) -> (x > 0?=w765:bool)
            n118 = local read "curX"() -> (w767:dbl)
            n119 = local read "curY"() -> (w766:dbl)
            n120 = control-ref of="CircleRadius"() -> ()  [unwired: 1 out]
            n121 = local read "ROI Descriptor COLOR"() -> (w759:T5)
            n122 = call "Ball ROI (SubVI).vi"("ROI Descriptor COLOR Mask"=w759, "divider (circle)"="divider (circle)", "curY"=w766, "curX"=w767, "Boolean"=w765) -> ("x1"=→"1x1 (circle)":i32, "y0"=→"1y0 (circle)":i32, "x0"=→"1x0 (circle)":i32, "ROI Descriptor COLOR Mask out"=w760:T5, "y1"=→"1y1 (circle)":i32)  [unwired: 2 in]
            n123 = local write "ROI Descriptor COLOR"(w760) -> ()
          }
          frame "(ball) Analyze color" {
            # "Color analyze"
            # "analyzed image buffer is\ncreated during the first\ncall of the Vision\nAssistant Express VI *only*\nwhen \"Create Destination\nImage\" option is enabled"
            # "Analyze image -- Analyze the webcam image with a Vision Assistant script."
            n124 = Unbundle By Name "Unbundle By Name"(w798) -> ("Color classes"=w792:i32[], "qsm.Webcam image ref"=w790:T8)
            n125 = call "Vision Assistant2"("Image In"=w790, "error in"=w787, "ROI Descriptor (Image Mask 1)"="ROI Descriptor COLOR", "ROI Descriptor (Color Classification 1)"="ROI Descriptor COLOR") -> ("Image Out"=w788:T8, "Classes (Color Classification 1)"=w789:string[])  [unwired: 21 in, 1 out]
            n126 = local read "(auto) balls counter"() -> (w791:i32)
            n127 = Index Array(array=w789, index=0) -> (element=w796:string)
            n128 = Decimal String To Number(string=w796) -> (number=w784:i32)  [unwired: 2 in, 1 out]
            "Color" <- w784
            n129 = Replace Array Subset(array=w792, new element=w784, index=w791) -> (w793:i32[])
            n130 = Bundle By Name "Bundle By Name"(cluster=w798, "qsm.Analyzed image ref"=w788, "Color class"=w784, "Color classes"=w793) -> (w797:T11)
            n131 = local read "1"() -> (w783:i32)
            n132 = local read "2"() -> (w782:i32)
            n133 = local read "3"() -> (w781:i32)
            n134 = local read "4"() -> (w780:i32)
            n135 = local read "5"() -> (w779:i32)
            n136 = Equal?(x=w783, y=w784) -> (x = y?=w774:bool)
            n137 = Equal?(x=w782, y=w784) -> (x = y?=w775:bool)
            n138 = Equal?(x=w781, y=w784) -> (x = y?=w776:bool)
            n139 = Equal?(x=w780, y=w784) -> (x = y?=w777:bool)
            n140 = Equal?(x=w779, y=w784) -> (x = y?=w778:bool)
            n141 = Build Array(w774, w775, w776, w777, w778) -> (w773:bool[])
            n142 = Or Array Elements(Boolean array=w773) -> (logical OR=→"Found Right Ball":bool)
          }
          frame "(ball) Align" {
            # "Align"
            # "Expansion State B"
          }
          frame "(ball) Wait" {
            # "Expansion State D"
            n143 = flat-sequence {
              frame #0 {
                n144 = Wait (ms)(milliseconds to wait="align accuracy") -> ()  [unwired: 1 out]
              }
              frame #1 {
                w815 = FALSE
                n145 = local write "Left-"(w815) -> ()
                n146 = local write "Left+"(w815) -> ()
                n147 = local write "Right+"(w815) -> ()
                n148 = local write "Right-"(w815) -> ()
              }
            }
            n149 = local read "X is in range"() -> (w812:bool)
            n150 = local read "Y is in range"() -> (w811:bool)
            n151 = And(x=w812, y=w811) -> (x .and. y?=w813:bool)
            n152 = case shown="True" w813 {
              selector: w813 -> [w817 w828]
              tunnel: w810 -> [w823 w830]
              tunnel: [w823 w830] -> w809
              tunnel: w808 -> [w822 w825]
              tunnel: [w820 w824] -> w807
              tunnel: w806 -> [w821 w829]
              tunnel: [w821 w829] -> _
              tunnel: w805 -> [_ _]
              tunnel: [w817 w828] -> w803
              frame False {
                n153 = Unbundle(T9 {"State"=enum."Align"} ("Shape - t, Color - f")) -> ("State"=w818:T1)
                n154 = local write "Found Right Ball"(FALSE ("Found Right Ball")) -> ()
                n155 = Bundle By Name(cluster=w822, "State"=w818) -> (w820:T9)
              }
              frame True {
                n156 = Unbundle(T9 {"State"=enum."Clear"} ("Shape - t, Color - f")) -> ("State"=w826:T1)
                n157 = Bundle By Name(cluster=w825, "State"=w826) -> (w824:T9)
              }
            }
            "Ready to Grab" <- w803
          }
          frame "(ball) Grab" {
            # "Expansion State E"
            n158 = call "(auto) Set Manip.vi"("G_upper bound"="M_UB_grab", "M_lower bound"="G_UB_grab", "error in (no error)"=w837) -> ("error out"=w835:errorcluster)  [unwired: 8 in]
            n159 = call "(auto) Set Manip.vi"("G_upper bound"="M_UB_pickUp", "M_lower bound"="G_UB_pickUp", "error in (no error)"=w835) -> ("error out"=w836:errorcluster)  [unwired: 8 in]
            "Grabbed" <- TRUE ("Grabbed")
          }
          frame "(pattern) Find Square" {
            # "analyzed image buffer is\ncreated during the first\ncall of the Vision\nAssistant Express VI *only*\nwhen \"Create Destination\nImage\" option is enabled"
            # "Expansion State F"
            n160 = Unbundle By Name "Unbundle By Name"(w842) -> ("qsm.Webcam image ref"=w859:T8)
            n161 = call "Vision Assistant3"("Image In"=w859, "error in"=w857) -> ("Image Out"=w855:T8, "Calibrated Matches (Geometric Matching 1)"=w854:T6[], "Number of Matches (Geometric Matching 1)"=→"Number of Matches (Geometric Matching 1)":i32)  [unwired: 22 in, 1 out]
            "Calibrated Matches (Geometric Matching 1)" <- w854
            n162 = Bundle By Name(cluster=w842, "qsm.Analyzed image ref"=w855) -> (w856:T11)
            n163 = Index Array(array=w854, index=0) -> (element=w852:T6)
            n164 = Unbundle By Name(w852) -> ("Position"=w851:cluster{"x":sgl, "y":sgl})
            n165 = Unbundle By Name(w851) -> ("x"=→"curX(p)":sgl)
            n166 = Unbundle By Name(w846) -> ("State"=w845:T1)
            n167 = Equal?(x=w845, y=T32."<mod>[P] comparing") -> (x = y?=w849:bool)
            n168 = case shown="True" w849 {
              tunnel: [w860 T32."(pattern) Align" ("Shape - t, Color - f")] -> w847
              tunnel: w845 -> [w860 _]
              frame False {
              }
              frame True {
              }
            }
            n169 = Bundle By Name(cluster=w846, "State"=w847) -> (w848:T9)
          }
          frame "(pattern) Calculate ROI" {
            # "Expansion State G"
          }
          frame "(pattern) Calc pattern indx" {
          }
          frame "Compare" {
            n170 = Unbundle By Name(w876) -> ("State"=w875:T1)
            n171 = Equal?(x=w875, y=T33."(mod) ball") -> (x = y?=w873:bool)
            n172 = Not(x=w873) -> (.not. x?=w872:bool)
            n173 = case shown="True" w872 {
              tunnel: w877 -> [w881 w887]
              frame False {
                n174 = local read "Ball number"() -> (w882:i32)
                n175 = control-ref of="ball match"() -> (w879:refnum<vi>)
                n176 = Unbundle By Name(w881) -> ("Color classes"=w880:i32[])
                n177 = Greater?(x=w882, y="Balls to remember") -> (0:w884:bool)
                n178 = call "(ball) Compare (SubVI).vi"("Boolean"=w884, "Balls to remember"="Balls to remember", "Ball number"=w882, "Color classes"=w880, "Boolean in"=w879) -> ("ball match"=→"ball match":bool)  [unwired: 6 in]
              }
              frame True {
                n179 = local read "CurDot"() -> (w885:T3)
                n180 = Greater?(x=w885, y="patterns to remember") -> (0:w889:bool)
                n181 = Unbundle By Name(w887) -> ("Pattern classes"=w886:i32[])
                n182 = case shown="True" w889 {
                  tunnel: "patterns to remember" -> [_ w893]
                  tunnel: w886 -> [_ w891]
                  tunnel: w885 -> [_ w890]
                  frame False {
                  }
                  frame True {
                    n183 = flat-sequence {
                      tunnel: w893 -> [w895]
                      tunnel: [w895] -> w892
                      tunnel: w892 -> [w898]
                      tunnel: w891 -> [w897]
                      tunnel: w890 -> [w896]
                      frame #0 {
                        n184 = local write "pattern match"(FALSE ("pattern match")) -> ()
                      }
                      frame #1 {
                        n185 = for {
                          N: w898 -> [_]
                          tunnel: w896 -> [w907]
                          tunnel: w897 -> [w901]
                          i -> [w903]
                          n186 = Increment(x=w903) -> (x+1=w902:i32)
                          n187 = Index Array(array=w901, index=w902) -> (element=w900:i32)
                          n188 = Index Array(array=w901, index=w907) -> (element=w899:i32)
                          n189 = Equal?(x=w900, y=w899) -> (x = y?=w906:bool)
                          n190 = local read "pattern match"() -> (w905:bool)
                          n191 = Not(x=w905) -> (.not. x?=w904:bool)
                          n192 = case shown="True" w904 {
                            tunnel: w906 -> [_ w908]
                            frame False {
                            }
                            frame True {
                              "pattern match" <- w908
                            }
                          }
                        }
                      }
                    }
                  }
                }
              }
            }
          }
          frame "(pattern) Analyze pattern" {
          }
          frame "(pattern) Align" {
            n193 = while {
              tunnel: w917 -> [w935]
              tunnel: [w933] -> w916
              shift-right: [w923] -> w914
              shift-left: w915 -> [w932]
              tunnel: w913 -> [w926]
              stop <- w927 stop-if-true
              n194 = flat-sequence {
                tunnel: [w944] -> w920
                tunnel: [w942] -> w936
                tunnel: [w943] -> w934
                tunnel: [w939] -> w925
                tunnel: w926 -> [w938]
                tunnel: w935 -> [w940]
                tunnel: [w937] -> w931
                tunnel: [w937] -> w921
                tunnel: w936 -> [w955]
                tunnel: w934 -> [w954]
                tunnel: [w954] -> w929
                tunnel: [w951] -> w928
                tunnel: [w950] -> w922
                tunnel: w921 -> [w950]
                tunnel: [w961] -> w933
                tunnel: w929 -> [w961]
                tunnel: w928 -> [w960]
                tunnel: [w959] -> w927
                tunnel: w924 -> [w958]
                tunnel: [w957] -> w923
                tunnel: w922 -> [w956]
                frame #0 {
                  n195 = local read "Angle for pattern (degrees)"() -> (w941:sgl)
                  n196 = call "full pattern analyze+remembering (SubVI).vi"("error in (no error)"=w940, "Angle (degrees)"=w941, "Patterns to remember"=w938) -> ("error out"=w943:errorcluster, 1:w946, "Pattern classes out"=w944:i32[], "Pattern"=w939:i32, 4:w945, 5:w937)  [unwired: 3 in]
                  n197 = Index Array(array=w945, index=0) -> (element=w948)
                  n198 = local write "Number of Matches (Geometric Matching 1)"(w946) -> ()
                  n199 = local write "Calibrated Matches (Geometric Matching 1)"(w945) -> ()
                  n200 = Unbundle By Name(w948) -> ("Position"=w947)
                  n201 = Unbundle By Name(w947) -> ("x"=w942)
                  n202 = local write "curX(p)"(w942) -> ()
                }
                frame #1 {
                  n203 = call "Pattern Align(SubVI).vi"("curX(p)"=w955, "defX(p)"="defX(p)", "Range(p)"="Range(p)") -> ("In Range?"=w951:bool)  [unwired: 8 in]
                  "In Range? (p)" <- w951
                }
                frame #2 {
                  n204 = case shown="True" w960 {
                    selector: w960 -> [w963 w991]
                    tunnel: [w963 w991] -> w959
                    tunnel: w958 -> [w962 w980]
                    tunnel: [w962 w973] -> w957
                    tunnel: w956 -> [_ w972]
                    frame False {
                    }
                    frame True {
                      n205 = local read "Number of Matches (Geometric Matching 1)"() -> (w989:i32)
                      n206 = Unbundle By Name(w980) -> ("qsm"=w966:T37, "ROI Descriptor (Image Mask 1)"=w970:T5, "Pattern classes"=w971:i32[])
                      n207 = local read "Calibrated Matches (Geometric Matching 1)"() -> (w988:T6[])
                      n208 = Unbundle(w970) -> ("Contours"=w977:T38)  [unwired: 1 out]
                      n209 = Greater Than 0?(x=w989) -> (x > 0?=w990:bool)
                      n210 = call "Pattern ROI (SubVI).vi"("divider"="divider (pattern)", "number of matches"=w990, "Calibrated Matches (Geometric Matching 1)"=w988, "Contours in"=w977) -> ("y1"=→"y1":i32, "x1"=→"x1":i32, "y0"=→"y0":i32, "Scale"=→"Scale":sgl, "x0"=→"x0":i32, "Contours out"=w969:T38)  [unwired: 2 in]
                      n211 = local read "CurDot"() -> (w979:T3)
                      n212 = To Long Integer(number=w979) -> (32bit integer=w978:i32)
                      n213 = Replace Array Subset(array=w977, new element=w969, index=0) -> (w975:T38)
                      n214 = Bundle(cluster=w970, "Contours"=w975) -> (w974:T5)  [unwired: 1 in]
                      n215 = call "(auto) Analyze pattern.vi"("Pattern classes"=w971, "Image In"=w972, "ROI Descriptor (Image Mask 1)"=w974, "pattern number"=w978) -> ("output array"=w964:i32[], "Image Out"=w965:T8, "Pattern"=→"Pattern":i32)  [unwired: 5 in]
                      n216 = Bundle(cluster=w970, "Contours"=w969) -> (w968:T5)  [unwired: 1 in]
                      n217 = Bundle(cluster=w966, "Analyzed image ref"=w965) -> (w967:T37)  [unwired: 2 in]
                      n218 = Bundle(cluster=w980, "qsm"=w967, "ROI Descriptor (Image Mask 1)"=w968, "Pattern classes"=w964) -> (w973:T11)  [unwired: 7 in]
                    }
                  }
                }
              }
              n219 = Bundle By Name(cluster=w932, "Session Out"=w925, "qsm.Webcam image ref"=w931) -> (w930:T11)
              n220 = local write "image display"(w920) -> ()
              n221 = Bundle By Name(cluster=w930, "qsm.Analyzed image ref"=w920) -> (w924:T11)
            }
          }
          frame "(pattern) Wait" {
            n222 = flat-sequence {
              tunnel: [w1001] -> w995
              tunnel: w994 -> [w1000]
              frame #0 {
                n223 = Wait (ms)(milliseconds to wait="align accuracy (p)") -> ()  [unwired: 1 out]
              }
              frame #1 {
                w999 = FALSE ("Right+")
                n224 = local write "Right+"(w999) -> ()
                n225 = local write "Right-"(w999) -> ()
                n226 = local write "Left+"(w999) -> ()
                n227 = local write "Left-"(w999) -> ()
              }
              frame #2 {
                n228 = local read "In Range? (p)"() -> (w1002:bool)
                n229 = Equal?(x=".Task", y=enum16{"Def", "<mod>[P]+tnl "}."<mod>[P]+tnl ") -> (x = y?=w1004:bool)
                n230 = And(x=w1002, y=w1004) -> (x .and. y?=w1003:bool)
                n231 = case shown="False" w1003 {
                  tunnel: [T32."(pattern) Align" ("Shape - t, Color - f") w1009] -> w1001
                  tunnel: w1000 -> [_ w1008]
                  frame False {
                  }
                  frame True {
                    n232 = Unbundle By Name(w1008) -> ("State"=w1009:T1)
                  }
                }
              }
            }
            n233 = Bundle By Name(cluster=w994, "State"=w995) -> (w996:T9)
          }
          frame "(pattern) states control" {
            n234 = flat-sequence {
              tunnel: w1011 -> [w1019]
              tunnel: w1011 -> [w1018]
              tunnel: [w1017] -> w1013
              frame #0 {
                n235 = Increment(x=",ctl num") -> (x+1=w1015:i32)
                n236 = local write ",ctl num"(w1015) -> ()
              }
              frame #1 {
                n237 = Unbundle By Name(w1019) -> ("State"=w1020:T1)
                n238 = case shown="\"<mod>[P] comparing\"" w1020 {
                  tunnel: w1018 -> [w1023 w1033 w1043 w1049 w1050 w1051 w1052 w1053 w1054 w1055 w1056 w1057 w1058 w1059 w1060 w1061 w1062 w1063 w1064 w1065 w1066 w1067 w1068 w1069 w1070 w1071 w1072 w1073 w1074 w1075 w1076 w1077]
                  tunnel: [w1022 w1032 w1043 w1049 w1050 w1051 w1052 w1053 w1054 w1055 w1056 w1057 w1058 w1059 w1060 w1061 w1062 w1063 w1064 w1065 w1066 w1067 w1068 w1069 w1070 w1071 w1072 w1073 w1074 w1075 w1076 w1077] -> w1017
                  frame "<mod>[P] remembering" {
                    n239 = local read ",ctl num"() -> (w1025:i32)
                    n240 = Greater?(x=w1025, y=3) -> (0:w1021:bool)
                    n241 = case shown="True" w1021 {
                      tunnel: w1023 -> [w1026 w1031]
                      tunnel: [w1026 w1030] -> w1022
                      frame False {
                      }
                      frame True {
                        n242 = Unbundle(T9 {"State"=enum."<mod>[P] go through tunnel"} ("Shape - t, Color - f")) -> ("State"=w1027:T1)
                        n243 = Bundle By Name(cluster=w1031, "State"=w1027) -> (w1030:T9)
                        n244 = local write ",ctl num"(0 ("ctl num")) -> ()
                      }
                    }
                  }
                  frame "<mod>[P] go through tunnel" {
                    n245 = local read ",ctl num"() -> (w1036:i32)
                    n246 = Greater?(x=w1036, y=1) -> (0:w1034:bool)
                    n247 = case shown="True" w1034 {
                      tunnel: w1033 -> [w1037 w1042]
                      tunnel: [w1037 w1041] -> w1032
                      frame False {
                      }
                      frame True {
                        n248 = Unbundle(T9 {"State"=enum."<mod>[P] comparing"}) -> ("State"=w1038:T1)
                        n249 = Bundle By Name(cluster=w1042, "State"=w1038) -> (w1041:T9)
                        n250 = local write ",ctl num"(0 (",ctl num")) -> ()
                      }
                    }
                  }
                  frame "<mod>[P] comparing" {
                    n251 = local read ",ctl num"() -> (w1045:i32)
                    n252 = Greater?(x=w1045, y=5) -> (0:w1046:bool)
                    n253 = case shown="True" w1046 {
                      frame False {
                      }
                      frame True {
                        n254 = local write ",ctl num"(0 (",ctl num")) -> ()
                        n255 = local write "Stop"(TRUE ("Stop")) -> ()
                      }
                    }
                  }
                  frame "(mod) ball" {
                  }
                  frame "Ball" {
                  }
                  frame "Other" {
                  }
                  frame "Clear" {
                  }
                  frame "(auto) Balls Analyze" {
                  }
                  frame "(auto) Ball Analyze" {
                  }
                  frame "Joystick control" {
                  }
                  frame "(mod) pattern" {
                  }
                  frame "Pattern" {
                  }
                  frame "(pattern) Align" {
                  }
                  frame "Align" {
                  }
                  frame "navx" {
                  }
                  frame "1" {
                  }
                  frame "2" {
                  }
                  frame "3" {
                  }
                  frame "4" {
                  }
                  frame "5" {
                  }
                  frame "6" {
                  }
                  frame "7" {
                  }
                  frame "8" {
                  }
                  frame "9" {
                  }
                  frame "10" {
                  }
                  frame "11" {
                  }
                  frame "12" {
                  }
                  frame "13" {
                  }
                  frame "(pattern) Align <loop>" {
                  }
                  frame "(ball) Align <loop>" {
                  }
                  frame "(auto) Recover Def Pos" {
                  }
                  frame "(auto) Go Back" {
                  }
                }
              }
            }
          }
          frame "navx" {
            n256 = disable-structure shown="Disabled" {
              disable-tunnel: w1080 -> [w1096 _]
              disable-tunnel: [w1095 _] -> w1079
              disable-tunnel: [w1092 _] -> w1078
              frame Disabled {
                n257 = call "sonic info (SubVI).vi"("error in (no error)"=w1096) -> ("error out"=w1095:errorcluster, "distance to the side"=w1094:u32)  [unwired: 9 in]
                "distance to the side" <- w1094
                n258 = Less Or Equal?(x=w1094, y=u32 7) -> (x <= y?=w1092:bool)
              }
              frame Enabled {
              }
            }
            n259 = disable-structure shown="Disabled" {
              disable-tunnel: _ -> [w1106 _]
              disable-tunnel: _ -> [w1105 _]
              disable-tunnel: [w1104 _] -> _
              disable-tunnel: [w1098 _] -> _
              disable-tunnel: [w1097 _] -> _
              frame Disabled {
                n260 = control-ref of="Left+"() -> (w1103:refnum<vi>)
                n261 = control-ref of="Left-"() -> (w1102:refnum<vi>)
                n262 = control-ref of="Right+"() -> (w1101:refnum<vi>)
                n263 = control-ref of="Right-"() -> (w1100:refnum<vi>)
                n264 = call "align.vi"(6:w1100, "I2C Ref Out"=w1106, "error in (no error)"=w1105, 9:w1101, 10:w1102, "Angle"=w1103) -> ("error out"=w1098:errorcluster, 1:w1097, "curAngle"=→"value Z":ext, "I2C Ref Out out"=w1104:T23)  [unwired: 2 in]
              }
              frame Enabled {
              }
            }
            n265 = control-ref of="L_PWM"() -> (w1088:refnum<vi>)
            n266 = control-ref of="R_PWM"() -> (w1087:refnum<vi>)
            n267 = call "fwd-navx (SubVI).vi"("error in (no error)"=w1079, "I2C Ref Out"=w1085, "R_PWM"=w1087, "L_PWM"=w1088) -> ("I2C Ref Out out"=w1089:T23, "value Z"=→"value Z 2":ext, "Right+"=w1084:bool, "Left+"=w1083:bool)  [unwired: 3 in, 1 out]
            n268 = Not(x=w1083) -> (.not. x?=w1082:bool)
            n269 = Not(x=w1084) -> (.not. x?=w1081:bool)
            n270 = local write "Left+"(w1083) -> ()
            n271 = local write "Left-"(w1082) -> ()
            n272 = local write "Right+"(w1084) -> ()
            n273 = local write "Right-"(w1081) -> ()
          }
          frame "stop motors" {
            n274 = flat-sequence {
              frame #0 {
                w1111 = TRUE ("Right+")
                n275 = local write "Left+"(w1111) -> ()
                n276 = local write "Left-"(w1111) -> ()
                n277 = local write "Right+"(w1111) -> ()
                n278 = local write "Right-"(w1111) -> ()
              }
              frame #1 {
                w1112 = FALSE ("Right+")
                n279 = local write "Left+"(w1112) -> ()
                n280 = local write "Left-"(w1112) -> ()
                n281 = local write "Right+"(w1112) -> ()
                n282 = local write "Right-"(w1112) -> ()
              }
            }
          }
          frame "(joystick) Joystick control" {
            n283 = shared-variable "My Computer\\KeyLibrary.lvlib\\Power"() -> (w1115:dbl)  [unwired: 1 in, 1 out]
            n284 = call "Joystick control (SubVI).vi"() -> ("G+"=w1121:bool, "M-"=w1123:bool, "M+"=w1122:bool, "G-"=w1120:bool, "Left+"=w1117:bool, "Right-"=w1116:bool, "Left-"=w1118:bool, "Right+"=w1119:bool)  [unwired: 4 in]
            n285 = local write "L_PWM"(w1115) -> ()
            n286 = local write "R_PWM"(w1115) -> ()
            n287 = local write "M-"(w1120) -> ()
            n288 = local write "G+"(w1122) -> ()
            n289 = local write "Right+"(w1119) -> ()
            n290 = local write "Right-"(w1116) -> ()
            n291 = local write "Left+"(w1117) -> ()
            n292 = local write "Left-"(w1118) -> ()
            n293 = local write "G-"(w1123) -> ()
            n294 = local write "M+"(w1121) -> ()
          }
          frame "_Timer" {
            n295 = Unbundle(T9 {"State"=enum."Align"} ("Shape - t, Color - f")) -> ("State"=w1126:T1)
            n296 = Bundle By Name(cluster=w1129, "State"=w1126) -> (w1128:T9)
          }
          frame "Setup manipulator" {
            (unwired) FALSE ("Release?")
            n297 = case shown="\"Align\", Default" "Manip state" {
              tunnel: ["G_UB_Align" w1144 w1146] -> w1134
              tunnel: ["M_UB_Align" w1145 w1146] -> w1135
              frame "Align", Default {
              }
              frame "Grab" {
                n298 = local read "M_UB_grab"() -> (w1145:i32)
                n299 = local read "G_UB_grab"() -> (w1144:i32)
              }
              frame "Release" {
                w1146 = 0
              }
            }
            n300 = call "Setup manipulator (SubVI).vi"("G_upper bound"=w1134, "M_lower bound"=w1135, "error in (no error)"=w1137, "M_Encoder Ref In"=w1139, "G_Encoder Ref In"=w1138) -> ()  [unwired: 10 in, 1 out]
          }
          frame "(auto) Count balls" {
            n301 = local read "Circles Calibrated (Shape Detection 1)"() -> (w1148:T4)
            n302 = call "(auto) Count balls (SubVI).vi"("error in"=w1147, "Circles Calibrated (Shape Detection 1)"=w1148) -> ("balls counter"=→"(auto) balls counter":i32)  [unwired: 8 in, 1 out]
          }
          frame "(auto) Analyze balls" {
            n303 = call "get.p.vi"("Session in"=w1154, "error in"=w1155) -> ("Image Out"=w1157:T8, "Session Out"=w1153:T12, "error out"=w1156:errorcluster)  [unwired: 23 in]
            "error out 2" <- w1156
            n304 = local read "(auto) balls counter"() -> (w1175:i32)
            n305 = call "Vision Assistant5"("Image In"=w1157, "error in"=w1156) -> ("error out"=w1159:errorcluster, "Circles Calibrated (Shape Detection 1)"=w1161:T4, "Number of Matches (Shape Detection 1)"=w1160:i32)  [unwired: 22 in, 1 out]
            "error out 3" <- w1159
            n306 = local write "Number of Matches (Shape Detection 1)"(w1160) -> ()
            n307 = local write "Circles Calibrated (Shape Detection 1)"(w1161) -> ()
            n308 = flat-sequence {
              tunnel: w1175 -> [w1190]
              tunnel: [w1189] -> w1174
              tunnel: [w1188] -> w1173
              tunnel: [w1187] -> w1169
              tunnel: [w1186] -> w1166
              tunnel: [w1185] -> w1165
              tunnel: w1161 -> [w1184]
              tunnel: w1160 -> [w1183]
              tunnel: w1159 -> [w1182]
              tunnel: w1157 -> [w1181]
              tunnel: w1166 -> [w1239]
              tunnel: w1165 -> [w1238]
              frame #0 {
                n309 = for {
                  N: w1190 -> [_]
                  tunnel: [w1202] -> w1189
                  tunnel: [w1201] -> w1188
                  tunnel: [w1197] -> w1187
                  tunnel: [w1196] -> w1186
                  tunnel: [w1195] -> w1185
                  tunnel: w1184 -> [w1193]
                  tunnel: w1183 -> [w1194]
                  tunnel: w1182 -> [w1192]
                  tunnel: w1181 -> [w1191]
                  i -> [w1199]
                  stop <- w1198 stop-if-true
                  n310 = flat-sequence {
                    tunnel: [w1222] -> w1202
                    tunnel: [w1219] -> w1201
                    tunnel: [w1211] -> w1200
                    tunnel: w1199 -> [_]
                    tunnel: [w1211] -> w1197
                    tunnel: [w1209] -> w1196
                    tunnel: [w1210] -> w1195
                    tunnel: w1193 -> [w1206]
                    tunnel: w1194 -> [w1205]
                    tunnel: w1192 -> [w1204]
                    tunnel: w1191 -> [w1203]
                    tunnel: w1200 -> [w1224]
                    tunnel: [w1223] -> w1198
                    frame #0 {
                      n311 = Index Array(array=w1206) -> (element=w1213:T36)  [unwired: 1 in]
                      n312 = Unbundle(w1213) -> ("Position"=w1212:cluster{"X":sgl, "Y":sgl}, "Radius"=w1208:dbl)  [unwired: 1 out]
                      n313 = local read "ROI Descriptor COLOR"() -> (w1221:T5)
                      n314 = Unbundle(w1212) -> ("X"=w1209:sgl, "Y"=w1210:sgl)
                      n315 = local read "divider (circle)"() -> (w1207:dbl)
                      n316 = Greater Than 0?(x=w1205) -> (x > 0?=w1214:bool)
                      n317 = call "Analyze ball (SubVI).vi"("ROI Descriptor COLOR Mask"=w1221, "Radius"=w1208, "Boolean"=w1214, "curX"=w1209, "curY"=w1210, "divider (circle)"=w1207, "Image In"=w1203, "error in"=w1204) -> ("Color"=w1211:i32, "Image Out"=w1222:T8, "error out"=w1219:errorcluster, "ROI Descriptor COLOR Mask out"=w1220:T5, "x0"=w1218:i32, "y0"=w1217:i32, "x1"=w1216:i32, "y1"=w1215:i32)  [unwired: 4 in]
                      n318 = local write "ROI Descriptor COLOR"(w1220) -> ()
                      n319 = local write "Color"(w1211) -> ()
                      n320 = local write "1x0 (circle)"(w1218) -> ()
                      n321 = local write "1x1 (circle)"(w1216) -> ()
                      n322 = local write "1y0 (circle)"(w1217) -> ()
                      n323 = local write "1y1 (circle)"(w1215) -> ()
                    }
                    frame #1 {
                      n324 = local read "1"() -> (w1229:i32)
                      n325 = local read "2"() -> (w1228:i32)
                      n326 = local read "3"() -> (w1227:i32)
                      n327 = local read "4"() -> (w1226:i32)
                      n328 = local read "5"() -> (w1225:i32)
                      n329 = Equal?(x=w1224, y=w1229) -> (x = y?=w1234:bool)
                      n330 = Equal?(x=w1224, y=w1228) -> (x = y?=w1233:bool)
                      n331 = Equal?(x=w1224, y=w1227) -> (x = y?=w1232:bool)
                      n332 = Equal?(x=w1224, y=w1226) -> (x = y?=w1231:bool)
                      n333 = Equal?(x=w1224, y=w1225) -> (x = y?=w1230:bool)
                      n334 = Build Array(w1234, w1233, w1232, w1231, w1230) -> (w1235:bool[])
                      n335 = Or Array Elements(Boolean array=w1235) -> (logical OR=w1223:bool)
                      n336 = local write "Found Right Ball"(w1223) -> ()
                    }
                  }
                }
                "error out 4" <- w1188
              }
              frame #1 {
                n337 = local read "Found Right Ball"() -> (w1240:bool)
                n338 = case shown="False" w1240 {
                  tunnel: [w1242 w1259] -> w1236
                  tunnel: [w1241 w1258] -> w1237
                  tunnel: w1239 -> [_ w1259]
                  tunnel: w1238 -> [_ w1258]
                  frame False {
                    n339 = local read "curY"() -> (w1241:dbl)
                    n340 = local read "curX"() -> (w1242:dbl)
                  }
                  frame True {
                    n341 = local read "Y is in range"() -> (w1251:bool)
                    n342 = local read "X is in range"() -> (w1250:bool)
                    n343 = local read "L_PWM"() -> (w1255:dbl)
                    n344 = local read "R_PWM"() -> (w1256:dbl)
                    n345 = call "Ball Align(SubVI).vi"("Align X - t, Y - f"="Align X - t, Y - f", "x is in range"=w1250, "y is in range"=w1251, "L_PWM"=w1255, "R_PWM"=w1256, "curX"=w1259, "defY"="defY", "curY"=w1258, "defX"="defX", "RangeY"="RangeY", "RangeX"="RangeX") -> ("x_is_in_range"=→"X is in range":bool, "y_is_in_range"=→"Y is in range":bool, "Ready to Grab()"=w1243:bool, "Align_X-t,Y-f"=w1252:bool, "L_PWM out"=w1253:dbl, "R_PWM out"=w1254:dbl)  [unwired: 10 in, 1 out]
                    n346 = local write "Ready to Grab"(w1243) -> ()
                    n347 = local write "Align X - t, Y - f"(w1252) -> ()
                    n348 = local write "R_PWM"(w1254) -> ()
                    n349 = local write "L_PWM"(w1253) -> ()
                  }
                }
                n350 = local write "curY"(w1237) -> ()
                n351 = local write "curX"(w1236) -> ()
              }
            }
            n352 = Unbundle By Name "Unbundle By Name"(w1168) -> ("Color classes"=w1171:i32[])
            n353 = local read "(auto) balls counter"() -> (w1172:i32)
            n354 = Replace Array Subset(array=w1171, new element=w1169, index=w1172) -> (w1170:i32[])
            n355 = local read "Ready to Grab"() -> (w1164:bool)
            n356 = Bundle By Name "Bundle By Name"(cluster=w1168, "qsm.Analyzed image ref"=w1174, "Color class"=w1169, "Color classes"=w1170, "Session Out"=w1153) -> (w1167:T11)
            n357 = case shown="True" w1164 {
              tunnel: [w1177 w1179] -> w1162
              tunnel: w1158 -> [w1178 _]
              frame False {
                n358 = Unbundle(w1178) -> ("State"=w1177:T1)
              }
              frame True {
                n359 = Unbundle(T9 {"State"=enum."Clear"} ("Shape - t, Color - f")) -> ("State"=w1179:T1)
              }
            }
            n360 = Bundle(cluster=w1158, "State"=w1162) -> (w1163:T9)
          }
          frame "(auto) Dot Controller" {
            # "here we should get and save: angle, L/R/M/G_enc's"
            # "here we should decide which of (auto) States we must use (DON'T USE 0)"
            n361 = local read "Grabbed"() -> (w1260:bool)
            n362 = case shown="False" w1260 {
              tunnel: w1269 -> [w1279 w1322]
              tunnel: w1268 -> [w1278 _]
              tunnel: w1267 -> [w1277 _]
              tunnel: w1266 -> [w1276 _]
              tunnel: w1265 -> [w1275 _]
              tunnel: w1264 -> [w1274 _]
              tunnel: [w1273 w1322] -> w1263
              tunnel: w1262 -> [w1272 w1323]
              tunnel: [w1271 w1320] -> w1261
              frame False {
                n363 = flat-sequence {
                  tunnel: w1278 -> [w1299]
                  tunnel: w1277 -> [w1286]
                  tunnel: w1276 -> [w1285]
                  tunnel: w1275 -> [w1284]
                  tunnel: w1274 -> [w1283]
                  tunnel: [w1282] -> _
                  tunnel: [w1298] -> w1281
                  tunnel: w1279 -> [w1300]
                  tunnel: w1281 -> [w1307]
                  tunnel: [w1307] -> w1280
                  tunnel: [w1313] -> w1273
                  tunnel: w1280 -> [w1313]
                  tunnel: w1272 -> [w1310]
                  tunnel: [w1308] -> w1271
                  frame #0 {
                    n364 = local read "Angles"() -> (w1296:dbl[])
                    n365 = local read "Left_enc"() -> (w1295:i32[])
                    n366 = local read "Right_enc"() -> (w1294:i32[])
                    n367 = local read "M_enc"() -> (w1293:i32[])
                    n368 = local read "G_enc"() -> (w1292:i32[])
                    n369 = Increment(x="CurDot") -> (x+1=w1297:T3)
                    n370 = local write "CurDot"(w1297) -> ()
                    n371 = call "(auto) SAVE.vi"("I2C Ref Out in"=w1300, "CurDot"=w1297, "Angles"=w1296, "Left_enc"=w1295, "Right_enc"=w1294, "M_enc"=w1293, "G_enc"=w1292, "error in (no error)"=w1299, "L_enc In"=w1286, "R_enc In"=w1285, "M_enc In"=w1284, "G_enc In"=w1283) -> ("I2C Ref Out out"=w1298:T23, "Angles out"=w1291:dbl[], "Left_enc out"=w1290:i32[], "Right_enc out"=w1289:i32[], "M_enc out"=w1288:i32[], "G_enc out"=w1287:i32[], "error out"=w1282:errorcluster)  [unwired: 9 in]
                    n372 = local write "Angles"(w1291) -> ()
                    n373 = local write "Left_enc"(w1290) -> ()
                    n374 = local write "Right_enc"(w1289) -> ()
                    n375 = local write "M_enc"(w1288) -> ()
                    n376 = local write "G_enc"(w1287) -> ()
                  }
                  frame #1 {
                    n377 = local read "States in total"() -> (w1306:i32)
                    n378 = local read "Dots of States"() -> (w1304:i32[][])
                    n379 = local read "Dots in total"() -> (w1303:i32)
                    n380 = local read "CurDot"() -> (w1305:T3)
                    n381 = call "(auto) Get State (SubVI).vi"("Dots in total"=w1303, "States in total"=w1306, "CurDot"=w1305, "Dots of States"=w1304) -> ("(auto) States"=w1302:T3)  [unwired: 7 in]
                    n382 = local write "(auto) States"(w1302) -> ()
                  }
                  frame #2 {
                    n383 = To Long Integer(number="(auto) States") -> (32bit integer=w1309:i32)
                    n384 = Greater Than 0?(x=w1309) -> (x > 0?=w1311:bool)
                    n385 = case shown="True" w1311 {
                      tunnel: w1310 -> [w1315 w1318]
                      tunnel: w1309 -> [_ w1317]
                      tunnel: [w1315 w1316] -> w1308
                      frame False {
                        n386 = local write "Stop"(TRUE ("Stop")) -> ()
                      }
                      frame True {
                        n387 = Bundle By Name(cluster=w1318, "State"=w1317) -> (w1316:T9)
                      }
                    }
                  }
                }
              }
              frame True {
                n388 = case shown="True" "At Def pos" {
                  tunnel: [w1324 w1326] -> w1319
                  frame False {
                    n389 = Unbundle(T9 {"State"=enum."(auto) Recover Def Pos"} ("Shape - t, Color - f")) -> ("State"=w1324:T1)
                  }
                  frame True {
                    n390 = Unbundle(T9 {"State"=enum."(auto) Go Back"} ("Shape - t, Color - f")) -> ("State"=w1326:T1)
                  }
                }
                n391 = Bundle By Name(cluster=w1323, "State"=w1319) -> (w1320:T9)
              }
            }
          }
          frame "(auto) Fwd (cm)" {
            n392 = call "movement forward by santimeters.vi"("I2C Ref in"=w1329, "error in (no error)"=w1331, "distance (cm)"=40.0) -> ("error out"=w1332:errorcluster, "I2C Ref out"=w1328:T23)  [unwired: 7 in]
          }
          frame "(auto) Turn (angle)" {
            n393 = call "rotate(NORMALNOE ROTATE).vi"("I2C Ref in"=w1336, "On/Off\nRight/Left"=FALSE ("On/Off\nRight/Left"), "error in (no error)"=w1339) -> ("error out"=w1338:errorcluster, "I2C Ref out"=w1335:T23)  [unwired: 7 in]
          }
          frame "(auto) Tnl (M2-M2.5)" {
            n394 = call "tunnel M2-M2.5.vi"("I2C Ref in"=w1343, "error in (no error)"=w1345) -> ("error out"=w1344:errorcluster, "I2C Ref Out"=w1342:T23)  [unwired: 8 in]
          }
          frame "(auto) Recover Def Pos" {
            n395 = local read "Right_enc"() -> (w1354:i32[])
            n396 = local read "Left_enc"() -> (w1355:i32[])
            n397 = local read "CurDot"() -> (w1353:T3)
            n398 = call "(auto) Recover def pos (SubVI).vi"("Right Encoder Ref In 2"=w1349, "Left Encoder Ref In"=w1350, "error in (no error)"=w1352, "CurDot"=w1353, "Left_enc"=w1355, "Right_enc"=w1354) -> ("error out"=w1351:errorcluster, "Recovered"=w1348:bool)  [unwired: 4 in]
            n399 = local write "At Def pos"(w1348) -> ()
          }
          frame "(auto) Go Back Controller" {
            n400 = local read "BackStates"() -> (w1362:enum16{"0", "1", "2", "3", "4", "5", "6", ""})
            n401 = local read "CurDot"() -> (w1363:T3)
            n402 = call "(auto) Go back controller.vi"("CurDot"=w1363, "BackStates"=w1362) -> ("BackState out"=w1361:enum16{"0", "1", "2", "3", "4", "5", "6", ""})  [unwired: 9 in]
            n403 = call "(auto) Go back Action.vi"("I2C Ref in"=w1360, "BackState"=w1361) -> ("I2C Ref Out"=w1359:T23)  [unwired: 9 in]
          }
          frame "Wait for button" {
            n404 = while {
              stop <- w1374 stop-if-true
              n405 = local read "Stop"() -> (w1376:bool)
              n406 = xnode "Button 2"() -> ("Value"=w1372:bool)  [unwired: 1 in, 1 out]
              n407 = Or(x="Next step", y=w1376) -> (x .or. y?=w1373:bool)
              n408 = Or(x=w1373, y=w1372) -> (x .or. y?=w1374:bool)
            }
            n409 = local write "Next step"(FALSE ("Look at ball")) -> ()
          }
        }
        n410 = xnode "Digital output (1 sample)"("Left+ (A/DIO5 (Pin 21))"="Left+", "Right+ (A/DIO7 (Pin 25))"="Right+", "Left- (A/DIO6 (Pin 23))"="Left-", "Right- (A/DIO13 (Pin 26))"="Right-", "error in (no error)"=w128) -> ("error out"=w177:errorcluster)
        n411 = xnode "Digital output (1 sample) 2"("G- (B/DIO7 (Pin 25))"="G-", "G+ (B/DIO13 (Pin 26))"="G+", "M+ (B/DIO5 (Pin 21))"="M+", "M- (B/DIO6 (Pin 23))"="M-", "error in (no error)"=w119) -> ("error out"=w176:errorcluster)
        n412 = Merge Errors(w177, w176) -> (w165:errorcluster)
        n413 = local read "ball match"() -> (w141:bool)
        n414 = local read "pattern match"() -> (w139:bool)
        n415 = Or(x=w141, y="ball = pattern?") -> (x .or. y?=w142:bool)
        n416 = Or(x=w142, y=w139) -> (x .or. y?=w140:bool)
        n417 = xnode "LED"("LED0"=w140, "LED1"=w140, "LED2"=w140, "LED3"=w140, "error in (no error)"=w165) -> ("error out"=w164:errorcluster)
        n418 = Unbundle(w91) -> ("State"=→"State":T1)
        n419 = Unbundle By Name(w90) -> ("Pattern classes"=w163:i32[], "Color classes"=w157:i32[])
        "Color classes" <- w157
        "Pattern classes" <- w163
        n420 = Merge Errors(w158, w164) -> (w179:errorcluster)
        n421 = local read "Number of Matches (Shape Detection 1)"() -> (w162:i32)
        n422 = local read "Ball number"() -> (w156:i32)
        n423 = Index Array(array=w163) -> (element=w143:i32)  [unwired: 1 in]
        n424 = Index Array(array=w157, index=w156) -> (element=w144:i32)
        n425 = Equal?(x=w144, y="1") -> (x = y?=→"1b":bool)
        n426 = Equal?(x=w144, y="2") -> (x = y?=→"2b":bool)
        n427 = Equal?(x=w144, y="3") -> (x = y?=→"3b":bool)
        n428 = Equal?(x=w144, y="4") -> (x = y?=→"4b":bool)
        n429 = Equal?(x=w144, y="5") -> (x = y?=→"5b":bool)
        n430 = Equal?(x=w143, y=w144) -> (x = y?=w159:bool)
        n431 = local write "ball = pattern?"(w159) -> ()
        n432 = Greater Than 0?(x=w162) -> (x > 0?=w161:bool)
        n433 = case shown="True" w161 {
          tunnel: [w225 w231] -> w87
          tunnel: w90 -> [w224 w231]
          frame False {
            n434 = Unbundle By Name(w224) -> ("Color classes"=w221:i32[])
            n435 = for {
              N: 5 -> [w229]
              tunnel: [w230] -> w223
              tunnel: w221 -> [w227]
              n436 = Decrement(x=w229) -> (x-1=w228:i32)
              n437 = Replace Array Subset(array=w227, new element=20, index=w228) -> (w230:i32[])
            }
            n438 = Bundle By Name(cluster=w224, "Color classes"=w223) -> (w225:T11)
          }
          frame True {
          }
        }
        n439 = Unbundle By Name(w87) -> ("Session Out"=w86:T12)
      }
    }
    frame #1 {
      w1413 = 0 ("(auto) balls counter")
      (unwired) TRUE ("Release?")
      w1427 = 0 ("G_upper bound")
      w1412 = FALSE ("X is in range")
      n440 = call "Setup manipulator (SubVI).vi"("G_upper bound"=w1427, "M_lower bound"=w1427, "error in (no error)"=w1428, "M_Encoder Ref In"=w1424, "G_Encoder Ref In"=w1423) -> ("error out"=w1422:errorcluster)  [unwired: 10 in]
      n441 = call <vilib>:"Close.vi"("error in (no error)"=w1428, "I2C Ref In"=w1432) -> ("error out"=w1416:errorcluster)  [unwired: 9 in]
      n442 = call <vilib>:"IMAQdx Close Camera.vi"("error in"=w1416, "Session In"=w1414) -> ("error out"=w1415:errorcluster)  [unwired: 9 in]
      n443 = call <vilib>:"Close.vi"("error in (no error)"=w1428, "PWM Ref In"=w1426) -> ("error out"=w1433:errorcluster)  [unwired: 9 in]
      n444 = call <vilib>:"Close.vi"("error in (no error)"=w1428, "PWM Ref In"=w1425) -> ("error out"=w1434:errorcluster)  [unwired: 9 in]
      n445 = call <vilib>:"Close.vi"("error in (no error)"=w1422, "Encoder Ref In"=w1424) -> ("error out"=w1429:errorcluster)  [unwired: 9 in]
      n446 = call <vilib>:"Close.vi"("error in (no error)"=w1422, "Encoder Ref In"=w1423) -> ("error out"=w1430:errorcluster)  [unwired: 9 in]
      n447 = call <vilib>:"Close.vi"("error in (no error)"=w1422, "Encoder Ref In"=w1420) -> ("error out"=w1419:errorcluster)  [unwired: 9 in]
      n448 = call <vilib>:"Close.vi"("error in (no error)"=w1422, "Encoder Ref In"=w1421) -> ("error out"=w1418:errorcluster)  [unwired: 9 in]
      n449 = Merge Errors(w1415, w1416, w1428, w1433, w1434, w1429, w1430, w1419, w1418) -> (w1435:errorcluster)
      n450 = local write "(auto) balls counter"(w1413) -> ()
      n451 = local write "Ball number"(1 ("Ball index")) -> ()
      n452 = call <vilib>:"Simple Error Handler.vi"("error in (no error)"=w1435) -> ("error out"=w1437:errorcluster)  [unwired: 4 in, 4 out]
      "error out" <- w1437
      n453 = local write "curY"(w1413) -> ()
      n454 = local write "curX"(w1413) -> ()
      n455 = local write "ball = pattern?"(w1412) -> ()
      n456 = local write "Ready to Grab"(w1412) -> ()
      n457 = local write "X is in range"(w1412) -> ()
      n458 = local write "R_PWM"("Def PWM") -> ()
      n459 = local write "Y is in range"(w1412) -> ()
      n460 = local write "L_PWM"("Def PWM") -> ()
      n461 = local write "At Def pos"(w1412) -> ()
      n462 = local write "Next step"(w1412) -> ()
      n463 = shared-variable "myRIO-1900\\vars.lvlib\\def Z"(ext -800.0 ("def Z")) -> ()  [unwired: 1 in, 1 out]
      n464 = local write "Grabbed"(w1412) -> ()
      n465 = local write "Right+"(w1412) -> ()
      n466 = local write "Right-"(w1412) -> ()
      n467 = local write "rotate"(w1412) -> ()
      n468 = local write "CurDot"(w1413) -> ()
      n469 = local write "Left+"(w1412) -> ()
      n470 = local write "Left-"(w1412) -> ()
      n471 = local write "Stop"(w1412) -> ()
      n472 = local write "M+"(w1412) -> ()
      n473 = local write "G+"(w1412) -> ()
      n474 = local write "M-"(w1412) -> ()
      n475 = local write "G-"(w1412) -> ()
    }
  }
  n476 = call <vilib>:"Reset myRIO.vi"("error in (no error)"=w63) -> ()  [unwired: 10 in, 1 out]
